vi "SpectrometerSpinCoater_v05.vi"() -> ()   [LabVIEW 2018]
uses:
  <instrlib>/Classes/CCD/Abstract_CCD/Abstract_CCD.lvclass
  TypDef/DeviceQueue_Action.ctl
  TypDef/DeviceQueue_TypeDef.ctl
  TypDef/DataQueue_Action.ctl
  TypDef/DataQueue_TypeDef.ctl
  <instrlib>/Classes/CCD/Avantes/Avantes.lvclass
  <vilib>/Utility/error.llb/DialogType.ctl
  <vilib>/Instr/_visa.llb/VISA Configure Serial Port (Instr).vi
  <vilib>/Analysis/NI_AALBase.lvlib
  <vilib>/Analysis/baseanly.llb/A x Vector.vi
  TypDef/TabControl.ctl
  C:/Program Files/National Instruments/LabVIEW 2018/instr.lib/Classes/CCD/Abstract_CCD/Abstract_CCD.lvclass
panel:
  out "Time.spin":refnum<file>
  out "Meas.spin":refnum<file>
  out "Arduino":bool
  out "NKT":bool
  out "Spectromter":bool
  in  "Abort Button":bool
  in  "Stop Button":bool
  in  "Tab Control":enum32{"Measure", "Settings"}(tab)=enum."Settings"
  in  "Spectra Count":u16
  in  "Measure Spectrum":bool
  out "Action":string
  in  "Preview":bool
  out "XY Graph":T1(graph)
  in  "Frames for Spectrometer":dbl=1.0
  in  "StartSpin_Button":bool
  out "Overall Time":dbl
  in  "Seconds after Spin Stop":dbl[unit]=0.5
  in  "Program Spin Coater\nSpeed (rpm)          Time (s)":dbl[][](array[numeric])
  in  "Record RefSpec":bool
  in  "Record_Darkspec":bool
  in  "Comments":string="Just for testing"
  in  "File Name":string="Temp"
  in  "Save Path":path=path "C:/Users/Timo/Desktop/SpinCoater/Measurement"
  in  "Seconds to Spin Start":dbl[unit]=1.0
  in  "Calculate Frames":bool=TRUE
  in  "Frames":i32
  out "Frame Rate":dbl[unit]
  in  "Integration Time":dbl[unit]=3e-05
  in  "StartMeasurement_Button":bool
  in  "Dividider Get Spectra":u32=1 min=1
  in  "Automatically \nadjust count":bool
  in  "Reset Count\nafter Spin Coating":bool
  in  "Speed":dbl
  in  "Milliseconds":dbl
  in  "Debug":bool
  in  "Port Arduino":refnum<visa-resource-name>="COM6"
  out "Error Arduino":bool caption="Error"
  in  "Init_Arduino":bool=TRUE caption="Init"
  out "Caption_Settings_Arduino":string="Arduino"
  out "Caption_Settings_NKT":string="NKT Laser"
  out "Error_Spectromter":bool caption="Error"
  in  "Init_Spectrometer":bool=TRUE caption="Init"
  out "Caption_Settings_Spectrometer":string="Spectromter"
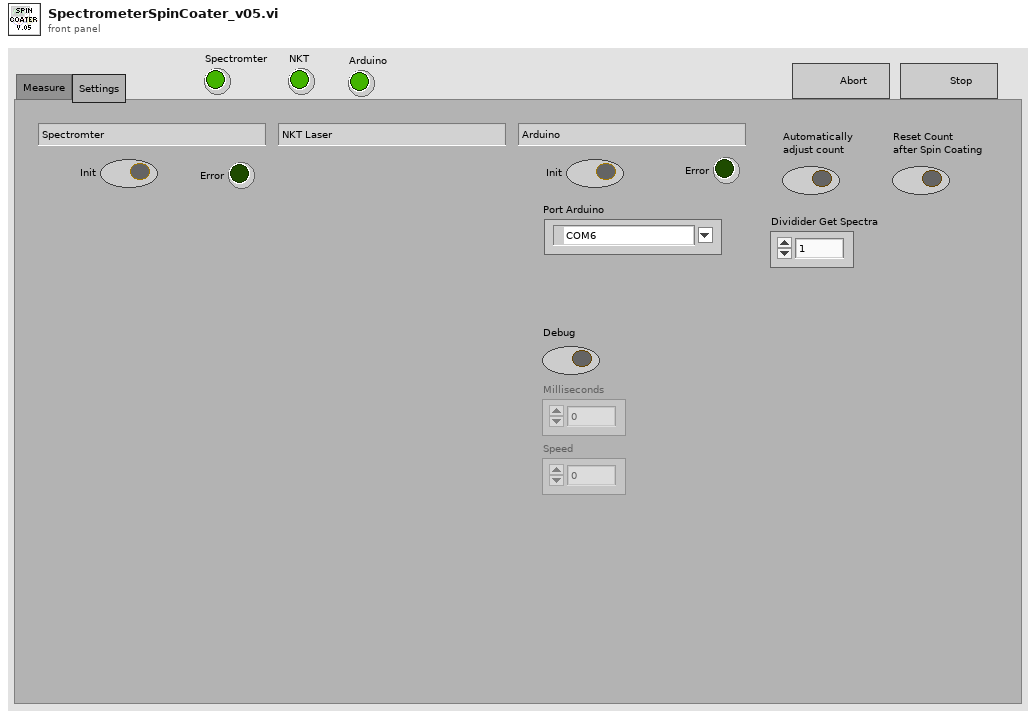
[diagram p1: front panel]
types:
  T1 = cluster{"Wavlength":dbl[unit][], "Image":dbl[]}[]
  T2 = cluster{"Dark":cluster{"Image":dbl[][][], "Frame Size":cluster{"F":i32, "Y":i32, "X":i32}}[], "Ref":cluster{"Image":dbl[][][], "Frame Size":cluster{"F":i32, "Y":i32, "X":i32}}[], "Wavlength":dbl[unit][], "spec":dbl[][]}
  T3 = cluster{"Port Arduino":refnum<visa-resource-name>, "Abstract_CCD.lvclass":refnum<class "Abstract_CCD.lvclass">}
  T4 = typedef "DataQueue_TypeDef.ctl" = cluster{"QueueAction":T5, "Data":cluster{"Image":dbl[][][], "Frame Size":cluster{"F":i32, "Y":i32, "X":i32}}[], "Data_Raw":cluster{"Image":dbl[][][], "Frame Size":cluster{"F":i32, "Y":i32, "X":i32}}[], "Data_Dark":cluster{"Image":dbl[][][], "Frame Size":cluster{"F":i32, "Y":i32, "X":i32}}[], "Data_Ref":cluster{"Image":dbl[][][], "Frame Size":cluster{"F":i32, "Y":i32, "X":i32}}[], "Device Information":string[], "Numeric Control":dbl, "Boolean":bool, "Wavelength":dbl[unit][], "Time":dbl[], "Time Stamp":timestamp, "Numeric Control 2":dbl, "TabControl":T6}
  T5 = typedef "DataQueue_Action.ctl" = enum16{"TimeOut", "Close_Program", "Abort", "Stop_Measurement", "Measure_InSituSpinCoating", "Measure_Spectrum", "Measure_SpectrumAdvanced", "Measure_SpectralStability", "Save_InSitu", "Save_SpectralStability", "Set_Ref", "Set_Dark", "Set_Wavelength", "Spectrometer_Measure", "Spectrometer_Preview", "Transfer_Settings"}
  T6 = typedef "TabControl.ctl" = enum16{"Measure", "Spectral Stability", "Settings"}
  T7 = typedef "DeviceQueue_TypeDef.ctl" = cluster{"QueueAction":T8, "Numeric 1":dbl, "Numeric 2":dbl, "Boolean 1":bool, "Boolean 2":bool, "Spin Program":dbl[][], "Spin Prg v07":cluster{"Speed (rpm)":dbl, "Time (s)":dbl, "Acc (rpm/s)":dbl}[], "Time Stamp":timestamp, "TabControl":T6}
  T8 = typedef "DeviceQueue_Action.ctl" = enum16{"TimeOut", "Wait", "Close_Program", "Abort", "Spectrometer_Init", "Spectrometer_Close", "Spectrometer_DeviceInformation", "Spectrometer_Measure", "Spectrometer_MeasureAdvanced", "Spectrometer_Preview", "Spectrometer_Abort", "Spectrometer_StartMeasurement", "Spectrometer_GetData", "Spectrometer_StopMeasurement", "Spectrometer_SetIntegrationTime", "Spectrometer_SetFrames", "Spectrometer_SetDarkspec", "Spectrometer_SetReference", "Spectrometer_SetTriggerMode", "Laser_Init", "Laser_Close", "Arduino_Init", "Arduino_Close", "Arduino_LoadProgram", "Arduino_StartProgram", "Arduino_SetSpeed", "Arduino_SetMillis", "Arduino_StopSpin", "Measure_InSitu", "Measure_Spectrum", "Measure_InSituAdvanced", "Measure_SpectralStability", "Measure_Stop"}
  T9 = typedef "DataQueue_Action.ctl" = enum16{"TimeOut", "Close_Program", "Stop_Measurement", "Measure_InSituSpinCoating", "Measure_Spectrum", "Save_Data", "Set_Ref", "Set_Dark", "Set_Wavelength", "Spectrometer_Measure", "Spectrometer_Preview", "Transfer_Settings"}
  T10 = enum16{"open", "replace", "create", "open or create", "replace or create", "replace or create with confirmation"}
  T11 = cluster{"Image":dbl[][][], "Frame Size":cluster{"F":i32, "Y":i32, "X":i32}}[]
  T12 = cluster{"Image":dbl[][][], "Frame Size":cluster{"F":i32, "Y":i32, "X":i32}}
  T13 = cluster{"Wavlength":dbl[unit][], "A x Vector":dbl[]}
  T14 = cluster{"Wavlength":dbl[unit][], "A x Vector":dbl[]}[]
  T15 = cluster{u16[][], u16[][], dbl[], "Numeric Control":dbl, "Numeric Control 2":dbl}
  T16 = typedef "DialogType.ctl" = u16
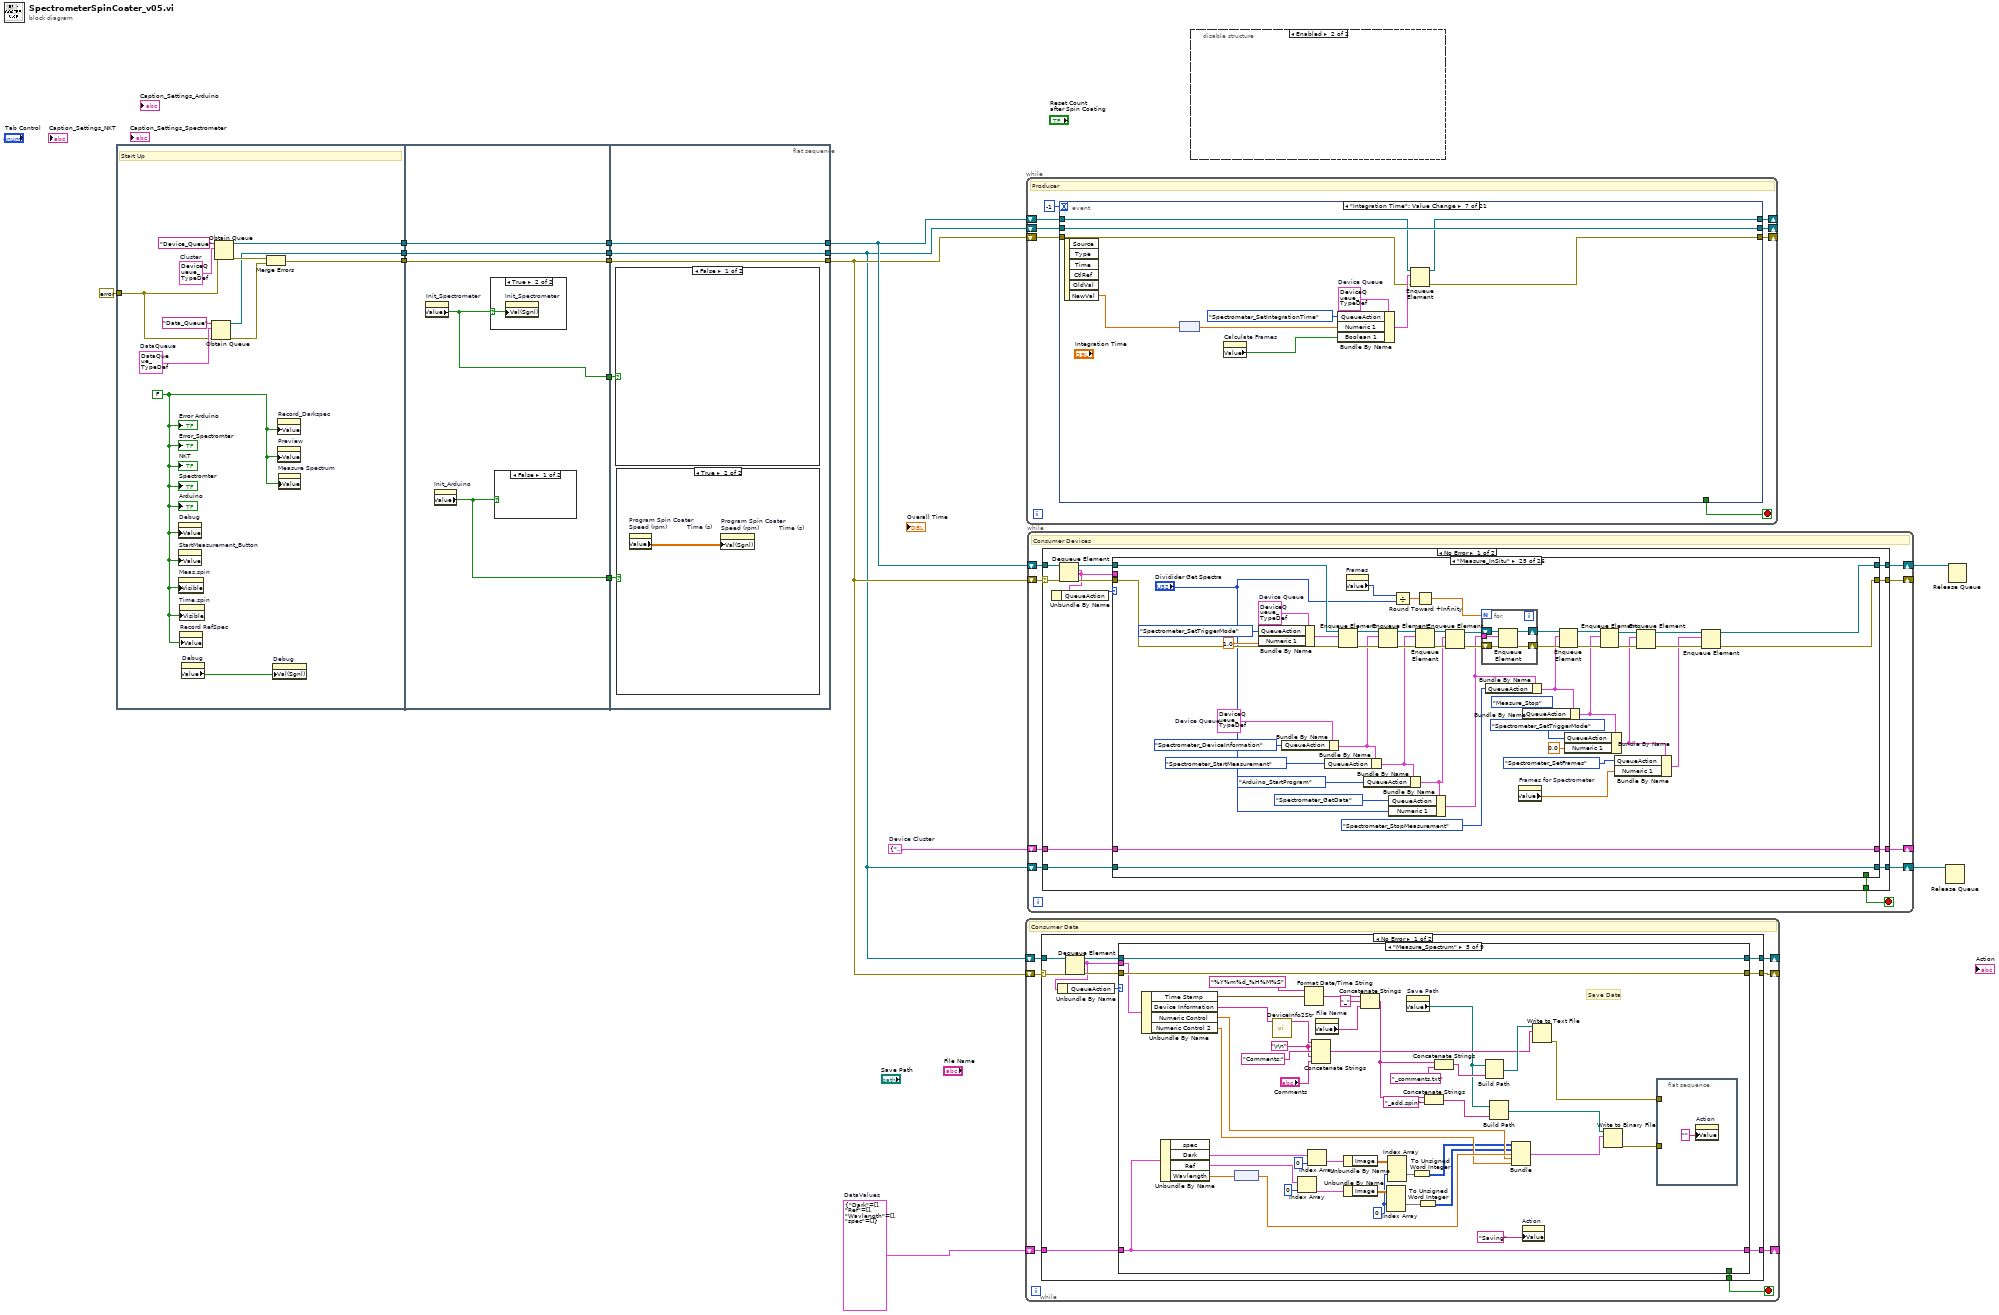
[diagram p0: block diagram]
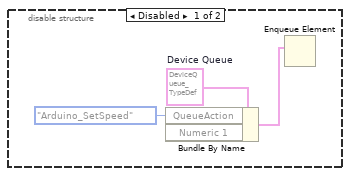
[diagram p2: hidden frame]
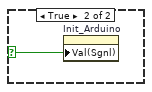
[diagram p3: hidden frame]
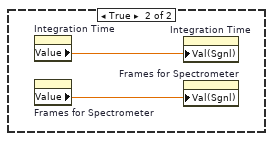
[diagram p6: hidden frame]
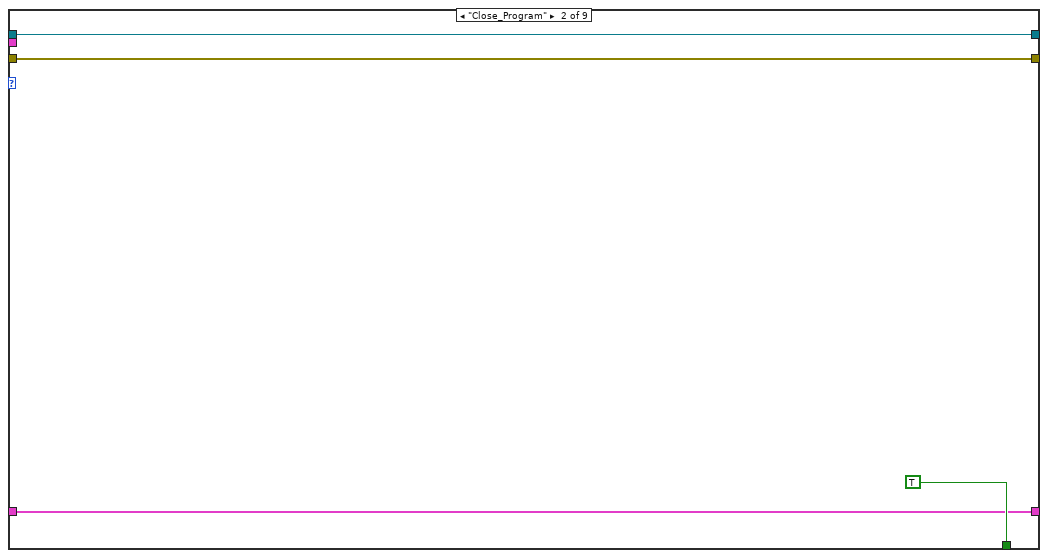
[diagram p8: hidden frame]
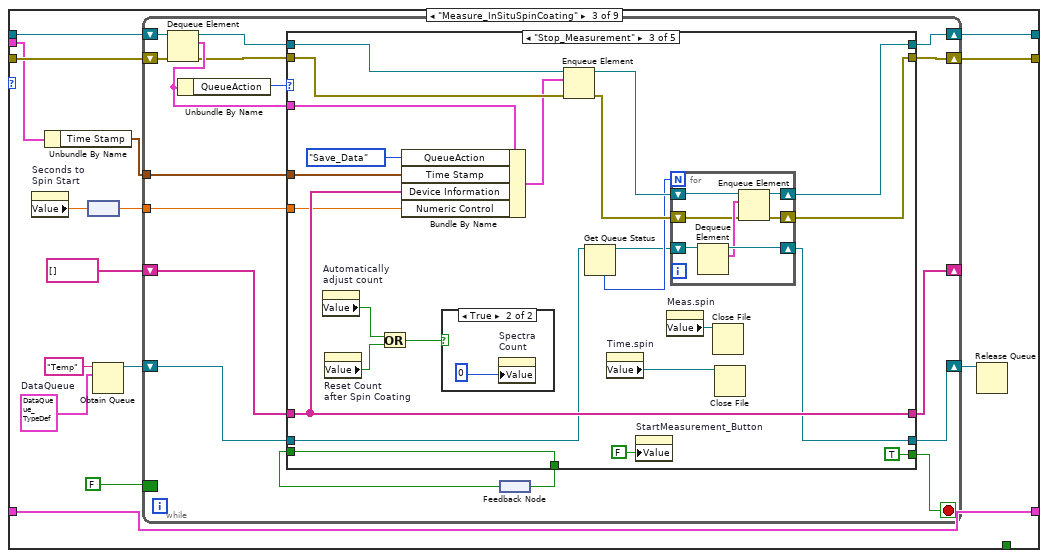
[diagram p9: hidden frame]
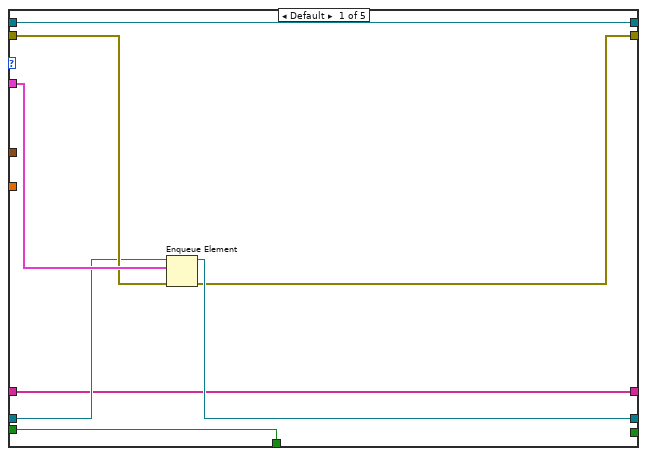
[diagram p10: hidden frame]
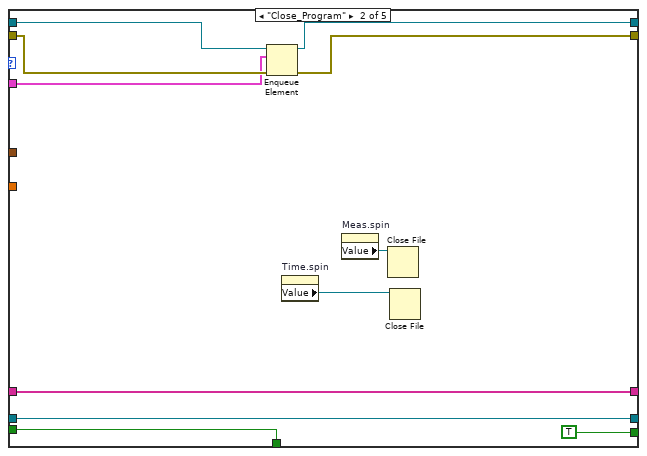
[diagram p11: hidden frame]
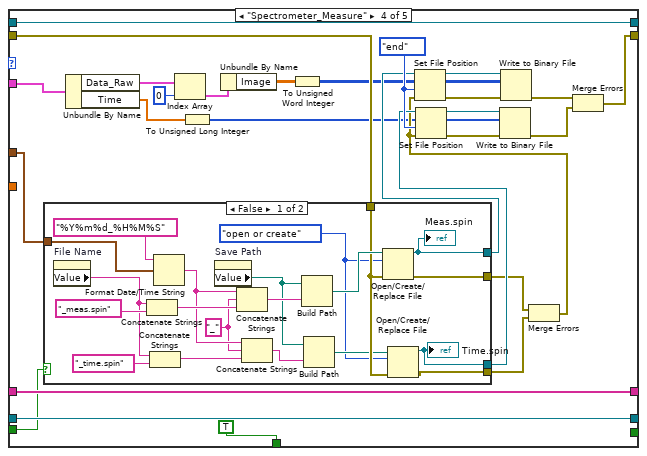
[diagram p13: hidden frame]
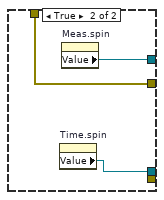
[diagram p14: hidden frame]
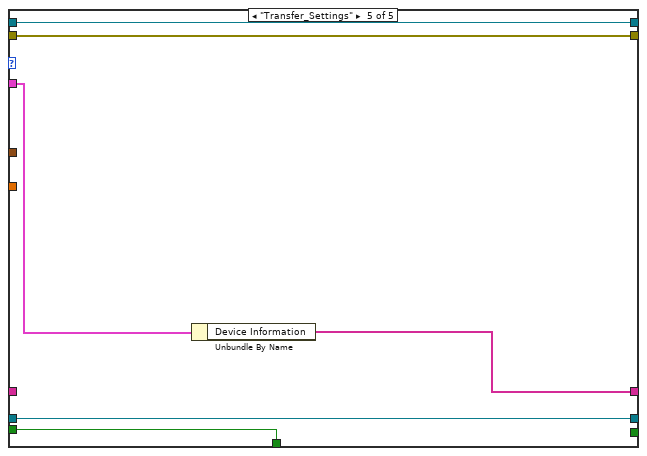
[diagram p15: hidden frame]
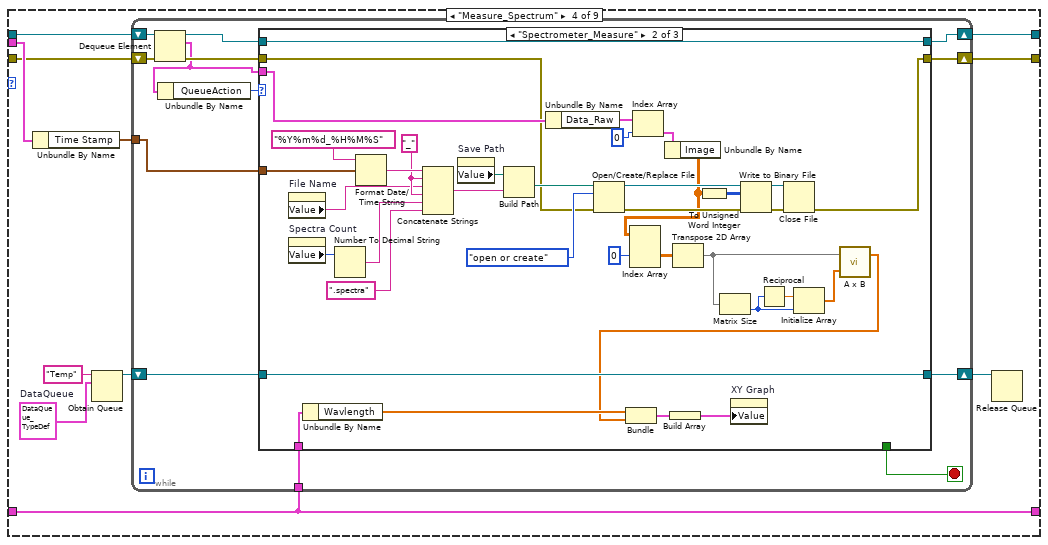
[diagram p16: hidden frame]
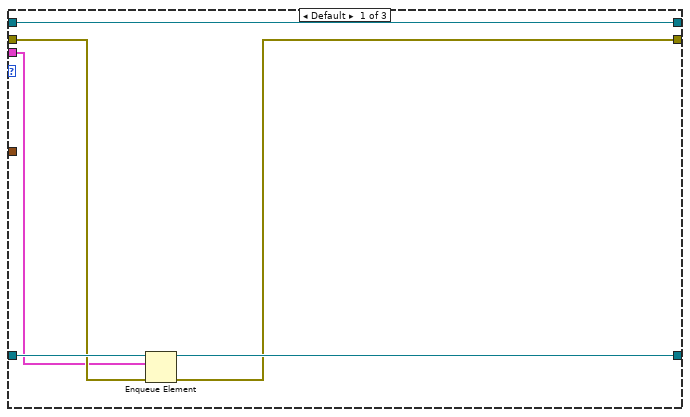
[diagram p17: hidden frame]
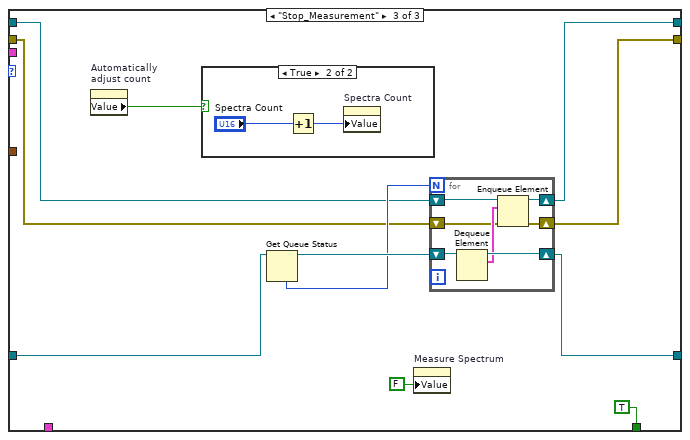
[diagram p18: hidden frame]
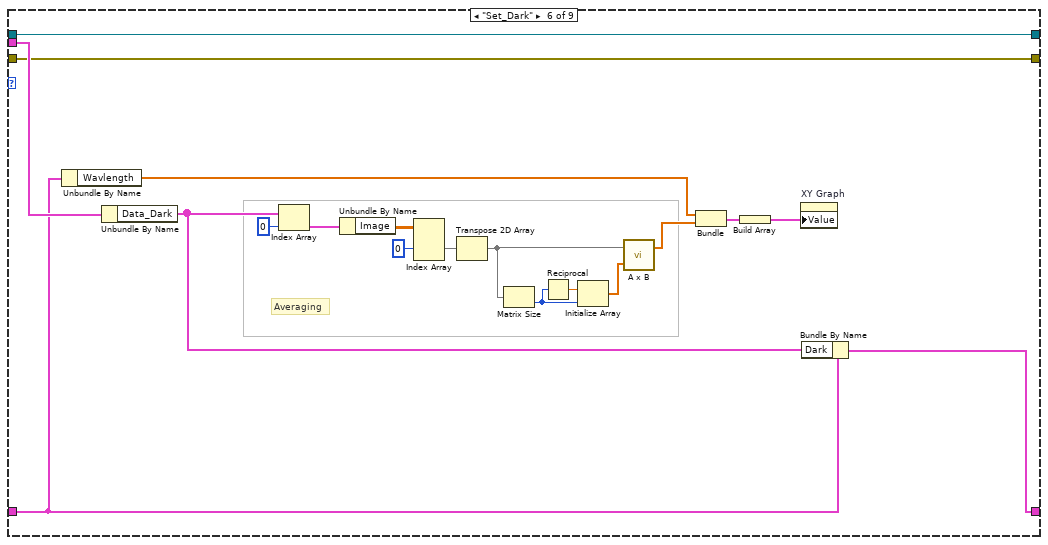
[diagram p20: hidden frame]
diagram:
  w6 = T2 {"Dark"=[], "Ref"=[], "Wavlength"=[], "spec"=[]}  # DataValues
  w11 = T3 {"Port Arduino"="", "Abstract_CCD.lvclass"=refnum}  # Device Cluster
  n1 = flat-sequence {
    tunnel: errorcluster {"status"=FALSE, "code"=0, "source"=""} ("error constant") -> [w23]
    tunnel: [w26] -> w15
    tunnel: [w20] -> w14
    tunnel: [w19] -> w13
    tunnel: w15 -> [w33]
    tunnel: w14 -> [w32]
    tunnel: w13 -> [w31]
    tunnel: [w33] -> w5
    tunnel: [w32] -> w4
    tunnel: [w31] -> w3
    tunnel: [w30] -> w2
    tunnel: [w29] -> w1
    tunnel: [w38] -> w8
    tunnel: [w39] -> w7
    tunnel: [w40] -> w12
    tunnel: w5 -> [w40]
    tunnel: w4 -> [w39]
    tunnel: w3 -> [w38]
    tunnel: w2 -> [w37]
    tunnel: w1 -> [w36]
    frame #0 {
      w24 = T4 {"QueueAction"=enum."TimeOut", "Data"=[], "Data_Raw"=[], "Data_Dark"=[], "Data_Ref"=[], "Device Information"=[], "Numeric Control"=0.0, "Boolean"=FALSE, "Wavelength"=[], "Time"=[], "Time Stamp"=timestamp(0 s since 1904-01-01), "Numeric Control 2"=0.0, "TabControl"=enum."Measure"}  # DataQueue
      w27 = T7 {"QueueAction"=enum."TimeOut", "Numeric 1"=0.0, "Numeric 2"=0.0, "Boolean 1"=FALSE, "Boolean 2"=FALSE, "Spin Program"=[], "Spin Prg v07"=[], "Time Stamp"=timestamp(0 s since 1904-01-01), "TabControl"=enum."Measure"}  # Cluster
      w18 = FALSE ("Error Arduino")
      # "Start Up"
      n2 = property on="Debug" class="Bool (strict)"("Value"=w18) -> ()  [unwired: 2 in, 2 out]
      n3 = property on="StartMeasurement_Button" class="Bool (strict)"("Value"=w18) -> ()  [unwired: 2 in, 2 out]
      n4 = property on="Meas.spin" class="Ref (strict)"("Visible"=w18) -> ()  [unwired: 2 in, 2 out]
      n5 = property on="Time.spin" class="Ref (strict)"("Visible"=w18) -> ()  [unwired: 2 in, 2 out]
      n6 = property on="Record RefSpec" class="Bool (strict)"("Value"=w18) -> ()  [unwired: 2 in, 2 out]
      n7 = property on="Debug" class="Bool (strict)"() -> ("Value"=w17:bool)  [unwired: 2 in, 2 out]
      n8 = Obtain Queue(name (unnamed)="Data_Queue", element data type=w24, error in (no error)=w23) -> (queue out=w20:refnum<queue>, error out=w21:errorcluster)  [unwired: 2 in, 1 out]
      n9 = Obtain Queue(name (unnamed)="Device_Queue", element data type=w27, error in (no error)=w23) -> (queue out=w26:refnum<queue>, error out=w22:errorcluster)  [unwired: 2 in, 1 out]
      n10 = Merge Errors(w22, w21) -> (w19:errorcluster)
      n11 = property on="Debug" class="Bool (strict)"("Val(Sgnl)"=w17) -> ()  [unwired: 2 in, 2 out]
      n12 = property on="Record_Darkspec" class="Bool (strict)"("Value"=w18) -> ()  [unwired: 2 in, 2 out]
      n13 = property on="Preview" class="Bool (strict)"("Value"=w18) -> ()  [unwired: 2 in, 2 out]
      n14 = property on="Measure Spectrum" class="Bool (strict)"("Value"=w18) -> ()  [unwired: 2 in, 2 out]
      "Error_Spectromter" <- w18
      "Error Arduino" <- w18
      "Spectromter" <- w18
      "NKT" <- w18
      "Arduino" <- w18
    }
    frame #1 {
      n15 = property on="Init_Spectrometer" class="Bool (strict)"() -> ("Value"=w30:bool)  [unwired: 2 in, 2 out]
      n16 = property on="Init_Arduino" class="Bool (strict)"() -> ("Value"=w29:bool)  [unwired: 2 in, 2 out]
      n17 = case shown="True" w30 {
        selector: w30 -> [_ w35]
        frame False {
        }
        frame True {
          n18 = property on="Init_Spectrometer" class="Bool (strict)"("Val(Sgnl)"=w35) -> ()  [unwired: 2 in, 2 out]
        }
      }
      n19 = case shown="False" w29 {
        selector: w29 -> [_ w34]
        frame False {
        }
        frame True {
          n20 = property on="Init_Arduino" class="Bool (strict)"("Val(Sgnl)"=w34) -> ()  [unwired: 2 in, 2 out]
        }
      }
    }
    frame #2 {
      n21 = case shown="False" w37 {
        frame False {
        }
        frame True {
          n22 = property on="Integration Time" class="DigNum (strict)"() -> ("Value"=w42:dbl[unit])  [unwired: 2 in, 2 out]
          n23 = property on="Frames for Spectrometer" class="DigNum (strict)"() -> ("Value"=w43:dbl)  [unwired: 2 in, 2 out]
          n24 = property on="Integration Time" class="DigNum (strict)"("Val(Sgnl)"=w42) -> ()  [unwired: 2 in, 2 out]
          n25 = property on="Frames for Spectrometer" class="DigNum (strict)"("Val(Sgnl)"=w43) -> ()  [unwired: 2 in, 2 out]
        }
      }
      n26 = case shown="True" w36 {
        frame False {
        }
        frame True {
          n27 = property on="Program Spin Coater\nSpeed (rpm)          Time (s)" class="Arr (strict)"() -> ("Value"=w41:dbl[][])  [unwired: 2 in, 2 out]
          n28 = property on="Program Spin Coater\nSpeed (rpm)          Time (s)" class="Arr (strict)"("Val(Sgnl)"=w41) -> ()  [unwired: 2 in, 2 out]
        }
      }
    }
  }
  n29 = while {
    shift-right: [w44] -> _
    shift-left: w8 -> [w50]
    shift-right: [w45] -> _
    shift-left: w7 -> [w49]
    shift-right: [w46] -> _
    shift-left: w6 -> [w48]
    stop <- w47 stop-if-true
    # "Consumer Data"
    n30 = case shown="No Error" w50 {
      selector: w50 -> [w61 w400]
      tunnel: w49 -> [w60 w401]
      tunnel: w48 -> [w58 w398]
      tunnel: [w57 _] -> w47
      tunnel: [w56 w398] -> w46
      tunnel: [w55 w401] -> w45
      tunnel: [w53 w399] -> w44
      frame No Error {
        n31 = Dequeue Element(queue=w60, error in (no error)=w61) -> (queue out=w54:refnum<queue>, element=w51:T4, error out=w52:errorcluster)  [unwired: 1 in, 1 out]
        n32 = Unbundle By Name(w51) -> ("QueueAction"=w59:T5)
        n33 = case shown="\"Measure_Spectrum\"" w59 {
          tunnel: w58 -> [w62 w67 w73 w209 w309 w352 w361 w383 w394]
          tunnel: [_ TRUE _ _ _ _ _ _ _] -> w57
          tunnel: [w62 w67 w73 w209 w309 w356 w375 w382 w394] -> w56
          tunnel: [w64 w66 w83 w215 w339 w357 w376 w379 w397] -> w55
          tunnel: w54 -> [w64 w66 w81 w217 w339 w357 w376 w379 w397]
          tunnel: [w63 w65 w82 w214 w338 w358 w377 w380 w396] -> w53
          tunnel: w52 -> [w63 w65 w80 w218 w338 w358 w377 w380 w396]
          tunnel: w51 -> [_ _ w75 w219 w325 w359 w378 w381 w395]
          frame "TimeOut", Default {
          }
          frame "Close_Program" {
          }
          frame "Measure_InSituSpinCoating" {
            w78 = T4 {"QueueAction"=enum."TimeOut", "Data"=[], "Data_Raw"=[], "Data_Dark"=[], "Data_Ref"=[], "Device Information"=[], "Numeric Control"=0.0, "Boolean"=FALSE, "Wavelength"=[], "Time"=[], "Time Stamp"=timestamp(0 s since 1904-01-01), "Numeric Control 2"=0.0, "TabControl"=enum."Measure"}  # DataQueue
            n34 = property on="Seconds to\nSpin Start" class="DigNum (strict)"() -> ("Value"=w70:dbl[unit])  [unwired: 2 in, 2 out]
            n35 = Unbundle By Name(w75) -> ("Time Stamp"=w74:timestamp)
            n36 = node(w70) -> (w69:dbl)
            n37 = Obtain Queue(name (unnamed)="Temp", element data type=w78) -> (queue out=w77:refnum<queue>)  [unwired: 3 in, 2 out]
            n38 = while {
              shift-right: [w91] -> w83
              shift-left: w81 -> [w100]
              shift-right: [w92] -> w82
              shift-left: w80 -> [w99]
              shift-right: [w93] -> w76
              shift-left: w77 -> [w94]
              tunnel: w74 -> [w87]
              shift-right: [w88] -> _
              shift-left: string[] [] ("Device Information") -> [w89]
              border: FALSE -> [_]
              tunnel: w69 -> [w84]
              stop <- w90 stop-if-true
              n39 = Dequeue Element(queue=w100, error in (no error)=w99) -> (queue out=w95:refnum<queue>, element=w97:T4, error out=w96:errorcluster)  [unwired: 1 in, 1 out]
              n40 = Unbundle By Name(w97) -> ("QueueAction"=w98:T5)
              n41 = feedback #1() -> (w86:bool)
              n42 = case shown="\"Stop_Measurement\"" w98 {
                tunnel: w97 -> [w108 w117 w142 w178 w207]
                tunnel: w96 -> [w107 w118 w139 w168 w204]
                tunnel: w95 -> [w103 w119 w138 w177 w205]
                tunnel: w94 -> [w106 w114 w133 w165 w208]
                tunnel: [w105 w114 w130 w165 w208] -> w93
                tunnel: [w104 w115 w129 w166 w204] -> w92
                tunnel: [w103 w116 w128 w177 w205] -> w91
                tunnel: [_ TRUE TRUE _ _] -> w90
                tunnel: w89 -> [w102 w112 w140 w163 _]
                tunnel: [w102 w112 w140 w163 w206] -> w88
                tunnel: w87 -> [_ _ w141 w179 _]
                tunnel: w86 -> [w101 w111 w127 w161 w203]
                tunnel: [w101 w111 w127 TRUE w203] -> w85
                tunnel: w84 -> [_ _ w124 _ _]
                frame Default {
                  n43 = Enqueue Element(queue=w106, element=w108, error in (no error)=w107) -> (queue out=w105:refnum<queue>, error out=w104:errorcluster)  [unwired: 1 in, 1 out]
                }
                frame "Close_Program" {
                  n44 = Enqueue Element(queue=w119, element=w117, error in (no error)=w118) -> (queue out=w116:refnum<queue>, error out=w115:errorcluster)  [unwired: 1 in, 1 out]
                  n45 = property on="Time.spin" class="Ref (strict)"() -> ("Value"=w109:refnum<file>)  [unwired: 2 in, 2 out]
                  n46 = property on="Meas.spin" class="Ref (strict)"() -> ("Value"=w110:refnum<file>)  [unwired: 2 in, 2 out]
                  n47 = Close File(refnum=w110) -> ()  [unwired: 1 in, 2 out]
                  n48 = Close File(refnum=w109) -> ()  [unwired: 1 in, 2 out]
                }
                frame "Stop_Measurement" {
                  n49 = property on="Automatically \nadjust count" class="Bool (strict)"() -> ("Value"=w121:bool)  [unwired: 2 in, 2 out]
                  n50 = property on="Reset Count\nafter Spin Coating" class="Bool (strict)"() -> ("Value"=w122:bool)  [unwired: 2 in, 2 out]
                  n51 = Or(x=w121, y=w122) -> (x .or. y?=w120:bool)
                  n52 = Bundle By Name(cluster=w142, "QueueAction"=DataQueue_Action."Save_Data", "Time Stamp"=w141, "Device Information"=w140, "Numeric Control"=w124) -> (w137:T4)
                  n53 = case shown="True" w120 {
                    frame False {
                    }
                    frame True {
                      n54 = property on="Spectra \nCount" class="DigNum (strict)"("Value"=u16 0 ("Spectra Count")) -> ()  [unwired: 2 in, 2 out]
                    }
                  }
                  n55 = Enqueue Element(queue=w138, element=w137, error in (no error)=w139) -> (queue out=w135:refnum<queue>, error out=w134:errorcluster)  [unwired: 1 in, 1 out]
                  n56 = Get Queue Status(queue=w133) -> (queue out=w131:refnum<queue>, # elements in queue=w132:i32)  [unwired: 2 in, 6 out]
                  n57 = property on="Time.spin" class="Ref (strict)"() -> ("Value"=w125:refnum<file>)  [unwired: 2 in, 2 out]
                  n58 = property on="StartMeasurement_Button" class="Bool (strict)"("Value"=FALSE ("StartMeasurement_Button")) -> ()  [unwired: 2 in, 2 out]
                  n59 = property on="Meas.spin" class="Ref (strict)"() -> ("Value"=w126:refnum<file>)  [unwired: 2 in, 2 out]
                  n60 = for {
                    N: w132 -> [_]
                    shift-right: [w150] -> w130
                    shift-left: w131 -> [w151]
                    shift-right: [w147] -> w128
                    shift-left: w135 -> [w148]
                    shift-right: [w145] -> w129
                    shift-left: w134 -> [w146]
                    n61 = Dequeue Element(queue=w151) -> (queue out=w150:refnum<queue>, element=w149:T4)  [unwired: 2 in, 2 out]
                    n62 = Enqueue Element(queue=w148, element=w149, error in (no error)=w146) -> (queue out=w147:refnum<queue>, error out=w145:errorcluster)  [unwired: 1 in, 1 out]
                  }
                  n63 = Close File(refnum=w126) -> ()  [unwired: 1 in, 2 out]
                  n64 = Close File(refnum=w125) -> ()  [unwired: 1 in, 2 out]
                }
                frame "Spectrometer_Measure" {
                  w164 = enum16{"start", "end", "current"}."end" ("from (0:start)")
                  n65 = case shown="False" w161 {
                    tunnel: w179 -> [w196 _]
                    tunnel: w168 -> [w191 w202]
                    tunnel: [w184 w202] -> w155
                    tunnel: [w183 _] -> w156
                    tunnel: [w182 w201] -> w158
                    tunnel: [w181 w200] -> w157
                    frame False {
                      w185 = T10."open or create" ("operation (0:open)")
                      w180 = "_" ("string")
                      n66 = property on="File Name" class="Str"() -> ("Value"=w194:string)  [unwired: 2 in, 2 out]
                      n67 = Concatenate Strings(w194, "_meas.spin" ("string")) -> (w197:string)
                      n68 = Concatenate Strings(w194, "_time.spin" ("string")) -> (w189:string)
                      n69 = Format Date/Time String(time format string (%c)="%Y%m%d_%H%M%S", seconds (now)=w196) -> (date/time string=w190:string)  [unwired: 1 in]
                      n70 = property on="Save Path" class="Path"() -> ("Value"=w187:path)  [unwired: 2 in, 2 out]
                      n71 = Concatenate Strings(w190, w180, w197) -> (w195:string)
                      n72 = Concatenate Strings(w190, w180, w189) -> (w188:string)
                      n73 = Build Path(base path=w187, name or relative path=w195) -> (appended path=w192:path)
                      n74 = Build Path(base path=w187, name or relative path=w188) -> (appended path=w186:path)
                      n75 = Open/Create/Replace File(file path (use dialog)=w192, error in=w191, operation (0:open)=w185) -> (refnum out=w182:refnum<file>, error out=w184:errorcluster)  [unwired: 3 in, 1 out]
                      "Meas.spin" <- w182
                      n76 = Open/Create/Replace File(file path (use dialog)=w186, error in=w191, operation (0:open)=w185) -> (refnum out=w181:refnum<file>, error out=w183:errorcluster)  [unwired: 3 in, 1 out]
                      "Time.spin" <- w181
                    }
                    frame True {
                      n77 = property on="Time.spin" class="Ref (strict)"() -> ("Value"=w200:refnum<file>)  [unwired: 2 in, 2 out]
                      n78 = property on="Meas.spin" class="Ref (strict)"() -> ("Value"=w201:refnum<file>)  [unwired: 2 in, 2 out]
                    }
                  }
                  n79 = Unbundle By Name(w178) -> ("Data_Raw"=w174:T11, "Time"=w167:dbl[])
                  n80 = Index Array(array=w174, index=0) -> (element=w173:T12)
                  n81 = To Unsigned Long Integer(number=w167) -> (unsigned 32bit integer=w153:u32[])
                  n82 = Unbundle By Name(w173) -> ("Image"=w171:dbl[][][])
                  n83 = To Unsigned Word Integer(number=w171) -> (unsigned 16bit integer=w152:u16[][][])
                  n84 = Merge Errors(w155, w156) -> (w154:errorcluster)
                  n85 = Set File Position(refnum=w158, from (0:start)=w164, error in=w154) -> (refnum out=w170:refnum<file>, error out=w169:errorcluster)  [unwired: 1 in]
                  n86 = Set File Position(refnum=w157, from (0:start)=w164, error in=w154) -> (refnum out=w176:refnum<file>, error out=w175:errorcluster)  [unwired: 1 in]
                  n87 = Write to Binary File(file (use dialog)=w176, data=w153, error in=w175) -> (error out=w159:errorcluster)  [unwired: 3 in, 2 out]
                  n88 = Write to Binary File(file (use dialog)=w170, data=w152, error in=w169) -> (error out=w160:errorcluster)  [unwired: 3 in, 2 out]
                  n89 = Merge Errors(w160, w159) -> (w166:errorcluster)
                }
                frame "Transfer_Settings" {
                  n90 = Unbundle By Name(w207) -> ("Device Information"=w206:string[])
                }
              }
              n91 = feedback-in #1(w85) -> ()
            }
            n92 = Release Queue(queue=w76) -> ()  [unwired: 2 in, 3 out]
          }
          frame "Measure_Spectrum" {
            w212 = T4 {"QueueAction"=enum."TimeOut", "Data"=[], "Data_Raw"=[], "Data_Dark"=[], "Data_Ref"=[], "Device Information"=[], "Numeric Control"=0.0, "Boolean"=FALSE, "Wavelength"=[], "Time"=[], "Time Stamp"=timestamp(0 s since 1904-01-01), "Numeric Control 2"=0.0, "TabControl"=enum."Measure"}  # DataQueue
            n93 = Unbundle By Name(w219) -> ("Time Stamp"=w216:timestamp)
            n94 = Obtain Queue(name (unnamed)="Temp", element data type=w212) -> (queue out=w211:refnum<queue>)  [unwired: 3 in, 2 out]
            n95 = while {
              shift-right: [w223] -> w215
              shift-left: w217 -> [w231]
              shift-right: [w224] -> w214
              shift-left: w218 -> [w232]
              tunnel: w216 -> [w221]
              shift-right: [w225] -> w210
              shift-left: w211 -> [w227]
              tunnel: w209 -> [w220]
              stop <- w222 stop-if-true
              n96 = Dequeue Element(queue=w231, error in (no error)=w232) -> (queue out=w229:refnum<queue>, element=w226:T4, error out=w228:errorcluster)  [unwired: 1 in, 1 out]
              n97 = Unbundle By Name(w226) -> ("QueueAction"=w230:T5)
              n98 = case shown="\"Spectrometer_Measure\"" w230 {
                tunnel: w229 -> [w233 w251 w282]
                tunnel: w228 -> [w236 w261 w281]
                tunnel: w227 -> [w238 w273 w284]
                tunnel: w226 -> [w234 w275 _]
                tunnel: [w237 w273 w280] -> w225
                tunnel: [w235 w252 w278] -> w224
                tunnel: [w233 w251 w279] -> w223
                tunnel: [_ _ TRUE] -> w222
                tunnel: w221 -> [_ w272 _]
                tunnel: w220 -> [_ w243 _]
                frame Default {
                  n99 = Enqueue Element(queue=w238, element=w234, error in (no error)=w236) -> (queue out=w237:refnum<queue>, error out=w235:errorcluster)  [unwired: 1 in, 1 out]
                }
                frame "Spectrometer_Measure" {
                  w269 = "_"
                  n100 = property on="File Name" class="Str"() -> ("Value"=w268:string)  [unwired: 2 in, 2 out]
                  n101 = property on="Spectra Count" class="DigNum (strict)"() -> ("Value"=w274:u16)  [unwired: 2 in, 2 out]
                  n102 = Unbundle By Name(w243) -> ("Wavlength"=w240:dbl[unit][])
                  n103 = Number To Decimal String(number=w274) -> (decimal integer string=w267:string)  [unwired: 1 in]
                  n104 = Format Date/Time String(time format string (%c)="%Y%m%d_%H%M%S", seconds (now)=w272) -> (date/time string=w270:string)  [unwired: 1 in]
                  n105 = Concatenate Strings(w270, w269, w268, w269, w267, ".spectra" ("string")) -> (w265:string)
                  n106 = property on="Save Path" class="Path"() -> ("Value"=w264:path)  [unwired: 2 in, 2 out]
                  n107 = Build Path(base path=w264, name or relative path=w265) -> (appended path=w263:path)
                  n108 = Unbundle By Name(w275) -> ("Data_Raw"=w258:T11)
                  n109 = Open/Create/Replace File(file path (use dialog)=w263, error in=w261, operation (0:open)=T10."open or create") -> (refnum out=w260:refnum<file>, error out=w259:errorcluster)  [unwired: 3 in, 1 out]
                  n110 = Index Array(array=w258, index=0) -> (element=w256:T12)
                  n111 = Unbundle By Name(w256) -> ("Image"=w244:dbl[][][])
                  n112 = Index Array(array=w244, index (dim 1)=0 ("disabled index (row)")) -> (element=w250:dbl[][])  [unwired: 2 in]
                  n113 = Transpose 2D Array(2D array=w250) -> (transposed array=w247:dbl[][])
                  n114 = To Unsigned Word Integer(number=w244) -> (unsigned 16bit integer=w255:u16[][][])
                  n115 = Matrix Size(0:w247) -> (2:w248:i32)  [unwired: 1 out]
                  n116 = Write to Binary File(file (use dialog)=w260, data=w255, error in=w259) -> (refnum out=w253:refnum<file>, error out=w254:errorcluster)  [unwired: 3 in, 1 out]
                  n117 = Reciprocal(x=w248) -> (1/x=w249:dbl)
                  n118 = Close File(refnum=w253, error in=w254) -> (error out=w252:errorcluster)  [unwired: 1 out]
                  n119 = Initialize Array(w249, w248) -> (w246:dbl[])
                  n120 = call-poly <vilib>:"A x B.vi"("Vector"=w246, "A"=w247) -> ("A x Vector"=w239:dbl[])  [unwired: 1 out]
                  n121 = Bundle("Wavlength"=w240, "A x Vector"=w239) -> (w242:T13)  [unwired: 1 in]
                  n122 = Build Array(w242) -> (w241:T14)
                  n123 = property on="XY Graph" class="XYGraph (strict)"("Value"=w241) -> ()  [unwired: 2 in, 2 out]
                }
                frame "Stop_Measurement" {
                  n124 = property on="Automatically \nadjust count" class="Bool (strict)"() -> ("Value"=w276:bool)  [unwired: 2 in, 2 out]
                  n125 = case shown="True" w276 {
                    frame False {
                    }
                    frame True {
                      n126 = Increment(x="Spectra Count") -> (x+1=w287:u16)
                      n127 = property on="Spectra Count" class="DigNum (strict)"("Value"=w287) -> ()  [unwired: 2 in, 2 out]
                    }
                  }
                  n128 = Get Queue Status(queue=w284) -> (queue out=w285:refnum<queue>, # elements in queue=w283:i32)  [unwired: 2 in, 6 out]
                  n129 = property on="Measure Spectrum" class="Bool (strict)"("Value"=FALSE ("Measure Spectrum")) -> ()  [unwired: 2 in, 2 out]
                  n130 = for {
                    N: w283 -> [_]
                    shift-right: [w294] -> w280
                    shift-left: w285 -> [w295]
                    shift-right: [w291] -> w279
                    shift-left: w282 -> [w292]
                    shift-right: [w289] -> w278
                    shift-left: w281 -> [w290]
                    n131 = Dequeue Element(queue=w295) -> (queue out=w294:refnum<queue>, element=w293:T4)  [unwired: 2 in, 2 out]
                    n132 = Enqueue Element(queue=w292, element=w293, error in (no error)=w290) -> (queue out=w291:refnum<queue>, error out=w289:errorcluster)  [unwired: 1 in, 1 out]
                  }
                }
              }
            }
            n133 = Release Queue(queue=w210) -> ()  [unwired: 2 in, 3 out]
          }
          frame "Measure_Spectrum" {
            w311 = "\r\n"
            w298 = 0 ("index (page)")
            # "Save Data"
            n134 = Unbundle By Name(w325) -> ("Time Stamp"=w323:timestamp, "Device Information"=w314:string[], "Numeric Control"=w308:dbl, "Numeric Control 2"=w307:dbl)
            n135 = Unbundle By Name(w309) -> ("Dark"=w335:T11, "Ref"=w333:T11, "Wavlength"=w337:dbl[unit][])  [unwired: 1 out]
            n136 = node(w337) -> (w326:dbl[])
            n137 = call "DeviceInfo2Str.vi"("Device Information"=w314) -> ("String"=w313:string)  [unwired: 10 in]
            n138 = Index Array(array=w333, index=0) -> (element=w331:T12)
            n139 = Format Date/Time String(time format string (%c)="%Y%m%d_%H%M%S", seconds (now)=w323) -> (date/time string=w322:string)  [unwired: 1 in]
            n140 = Index Array(array=w335, index=0) -> (element=w332:T12)
            n141 = Concatenate Strings(w313, w311, "Comments:" ("string"), w311, "Comments") -> (w306:string)
            n142 = property on="File Name" class="Str"() -> ("Value"=w304:string)  [unwired: 2 in, 2 out]
            n143 = Unbundle By Name(w332) -> ("Image"=w330:dbl[][][])
            n144 = Unbundle By Name(w331) -> ("Image"=w329:dbl[][][])
            n145 = Concatenate Strings(w322, "_" ("string"), w304) -> (w320:string)
            n146 = Index Array(array=w329, index (dim 1)=w298) -> (element=w327:dbl[][])  [unwired: 2 in]
            n147 = Index Array(array=w330, index (dim 1)=w298) -> (element=w328:dbl[][])  [unwired: 2 in]
            n148 = property on="Save Path" class="Path"() -> ("Value"=w303:path)  [unwired: 2 in, 2 out]
            n149 = To Unsigned Word Integer(number=w328) -> (unsigned 16bit integer=w297:u16[][])
            n150 = To Unsigned Word Integer(number=w327) -> (unsigned 16bit integer=w296:u16[][])
            n151 = Concatenate Strings(w320, "_add.spin" ("string")) -> (w318:string)
            n152 = Concatenate Strings(w320, "_comments.txt" ("string")) -> (w317:string)
            n153 = Build Path(base path=w303, name or relative path=w317) -> (appended path=w316:path)
            n154 = Build Path(base path=w303, name or relative path=w318) -> (appended path=w302:path)
            n155 = Bundle(w297, w296, w326, "Numeric Control"=w308, "Numeric Control 2"=w307) -> (w301:T15)  [unwired: 1 in]
            n156 = property on="Action" class="Str"("Value"="Saving" ("Action")) -> ()  [unwired: 2 in, 2 out]
            n157 = Write to Text File(file (use dialog)=w316, text=w306) -> (error out=w300:errorcluster)  [unwired: 2 in, 2 out]
            n158 = Write to Binary File(file (use dialog)=w302, data=w301) -> (error out=w299:errorcluster)  [unwired: 4 in, 2 out]
            n159 = flat-sequence {
              tunnel: w300 -> [_]
              tunnel: w299 -> [_]
              frame #0 {
                n160 = property on="Action" class="Str"("Value"="" ("Action")) -> ()  [unwired: 2 in, 2 out]
              }
            }
          }
          frame "Set_Dark" {
            # "Averaging"
            n161 = Unbundle By Name(w352) -> ("Wavlength"=w351:dbl[unit][])
            n162 = Unbundle By Name(w359) -> ("Data_Dark"=w349:T11)
            n163 = Index Array(array=w349, index=0) -> (element=w354:T12)
            n164 = Unbundle By Name(w354) -> ("Image"=w348:dbl[][][])
            n165 = Index Array(array=w348, index (dim 1)=0 ("disabled index (row)")) -> (element=w346:dbl[][])  [unwired: 2 in]
            n166 = Transpose 2D Array(2D array=w346) -> (transposed array=w343:dbl[][])
            n167 = Matrix Size(0:w343) -> (2:w344:i32)  [unwired: 1 out]
            n168 = Reciprocal(x=w344) -> (1/x=w345:dbl)
            n169 = Initialize Array(w345, w344) -> (w342:dbl[])
            n170 = call-poly <vilib>:"A x B.vi"("Vector"=w342, "A"=w343) -> ("A x Vector"=w341:dbl[])  [unwired: 1 out]
            n171 = Bundle("Wavlength"=w351, "A x Vector"=w341) -> (w353:T13)  [unwired: 1 in]
            n172 = Build Array(w353) -> (w350:T14)
            n173 = property on="XY Graph" class="XYGraph (strict)"("Value"=w350) -> ()  [unwired: 2 in, 2 out]
            n174 = Bundle By Name(cluster=w352, "Dark"=w349) -> (w356:T2)
          }
          frame "Set_Ref" {
            # "Averaging"
            n175 = Unbundle By Name(w361) -> ("Wavlength"=w360:dbl[unit][])
            n176 = Unbundle By Name(w378) -> ("Data_Ref"=w365:T11)
            n177 = Index Array(array=w365, index=0) -> (element=w373:T12)
            n178 = Unbundle By Name(w373) -> ("Image"=w372:dbl[][][])
            n179 = Index Array(array=w372, index (dim 1)=0 ("disabled index (row)")) -> (element=w370:dbl[][])  [unwired: 2 in]
            n180 = Transpose 2D Array(2D array=w370) -> (transposed array=w367:dbl[][])
            n181 = Matrix Size(0:w367) -> (2:w368:i32)  [unwired: 1 out]
            n182 = Reciprocal(x=w368) -> (1/x=w369:dbl)
            n183 = Initialize Array(w369, w368) -> (w366:dbl[])
            n184 = call-poly <vilib>:"A x B.vi"("Vector"=w366, "A"=w367) -> ("A x Vector"=w362:dbl[])  [unwired: 1 out]
            n185 = Bundle("Wavlength"=w360, "A x Vector"=w362) -> (w364:T13)  [unwired: 1 in]
            n186 = Build Array(w364) -> (w363:T14)
            n187 = Bundle By Name(cluster=w361, "Ref"=w365) -> (w375:T2)
            n188 = property on="XY Graph" class="XYGraph (strict)"("Value"=w363) -> ()  [unwired: 2 in, 2 out]
          }
          frame "Set_Wavelength" {
            n189 = Unbundle By Name(w381) -> ("Wavelength"=w384:dbl[unit][])
            n190 = Bundle By Name(cluster=w383, "Wavlength"=w384) -> (w382:T2)
          }
          frame "Spectrometer_Preview" {
            w389 = 0 ("index (page)")
            n191 = Unbundle By Name(w395) -> ("Data_Raw"=w393:T11)
            n192 = Unbundle By Name(w394) -> ("Wavlength"=w388:dbl[unit][])
            n193 = Index Array(array=w393, index=0) -> (element=w391:T12)
            n194 = Unbundle By Name(w391) -> ("Image"=w390:dbl[][][])
            n195 = Index Array(array=w390, index (dim 0)=w389, index (dim 1)=w389) -> (element=w387:dbl[])  [unwired: 1 in]
            n196 = Bundle("Wavlength"=w388, "Image"=w387) -> (w386:cluster{"Wavlength":dbl[unit][], "Image":dbl[]})  [unwired: 1 in]
            n197 = Build Array(w386) -> (→"XY Graph":T1)
          }
        }
      }
      frame Error {
        w403 = T16 4 items=["no dialog", "OK message", "continue or stop message", "OK message + warnings", "continue/stop + warnings"] ("type of dialog (OK msg:1)")
        n198 = call <vilib>:"General Error Handler.vi"("type of dialog (OK msg:1)"=w403, "error in (no error)"=w400) -> ("error out"=w402:errorcluster)  [unwired: 9 in, 4 out]
        n199 = call <vilib>:"Clear Errors.vi"("error in (no error)"=w402) -> ("error out"=w399:errorcluster)  [unwired: 5 in, 1 out]
      }
    }
  }
  n200 = while {
    shift-right: [w406] -> _
    shift-left: w12 -> [w404]
    shift-right: [w409] -> _
    shift-left: w7 -> [w410]
    shift-right: [w407] -> _
    shift-left: w8 -> [w408]
    stop <- w405 stop-if-true
    # "Producer"
    n201 = event shown="[6] \"Integration Time\": Value Change" {
      selector: _ -> [_ _ _ _ _ _ _ _ _ _ _ _ _ _ _ _ _ _ _ _ _]
      dyn-events: _ -> [_ _ _ _ _ _ _ _ _ _ _ _ _ _ _ _ _ _ _ _ _]
      timeout: -1 -> [_ _ _ _ _ _ _ _ _ _ _ _ _ _ _ _ _ _ _ _ _]
      tunnel: w410 -> [w413 w428 w432 w444 w457 w472 w484 w495 w498 w505 w524 w531 w540 w548 w563 w573 w582 w590 w595 w602 w614]
      tunnel: [w413 w425 w432 w444 w457 w472 w484 w495 w498 w505 w524 w531 w540 w547 w563 w573 w582 w590 w595 w600 w614] -> w409
      tunnel: w408 -> [w412 w427 w434 w442 w454 w471 w482 w490 w497 w502 w522 w530 w538 w554 w560 w572 w581 w589 w594 w607 w615]
      tunnel: [w412 w421 w431 w438 w453 w469 w480 w489 w497 w500 w521 w528 w537 w546 w561 w569 w578 w589 w594 w607 w615] -> w407
      tunnel: w404 -> [w414 w429 w435 w443 w456 w473 w483 w492 w499 w503 w525 w532 w541 w556 w564 w574 w583 w591 w596 w608 w613]
      tunnel: [w414 w426 w433 w439 w455 w470 w481 w491 w499 w504 w523 w529 w539 w555 w562 w570 w579 w591 w593 w606 w613] -> w406
      tunnel: [_ TRUE _ _ _ _ _ _ _ _ _ _ _ _ _ _ _ _ _ _ _] -> w405
      event Timeout {
        n202 = event-data() -> ()  [unwired: 1 in, 3 out]
      }
      event "Stop Button": Value Change {
        w417 = T4 {"QueueAction"=enum."TimeOut", "Data"=[], "Data_Raw"=[], "Data_Dark"=[], "Data_Ref"=[], "Device Information"=[], "Numeric Control"=0.0, "Boolean"=FALSE, "Wavelength"=[], "Time"=[], "Time Stamp"=timestamp(0 s since 1904-01-01), "Numeric Control 2"=0.0, "TabControl"=enum."Measure"}  # DataQueue
        w420 = T7 {"QueueAction"=enum."TimeOut", "Numeric 1"=0.0, "Numeric 2"=0.0, "Boolean 1"=FALSE, "Boolean 2"=FALSE, "Spin Program"=[], "Spin Prg v07"=[], "Time Stamp"=timestamp(0 s since 1904-01-01), "TabControl"=enum."Measure"}  # Device Queue
        n203 = event-data() -> ()  [unwired: 1 in, 6 out]
        n204 = Bundle By Name(cluster=w420, "QueueAction"=DeviceQueue_Action."Close_Program") -> (w418:T7)
        n205 = Enqueue Element(queue=w429, element=w418, error in (no error)=w427) -> (queue out=w426:refnum<queue>, error out=w422:errorcluster)  [unwired: 1 in, 1 out]
        n206 = Bundle By Name(cluster=w417, "QueueAction"=DataQueue_Action."Close_Program") -> (w415:T4)
        n207 = Enqueue Element(queue=w428, element=w415, error in (no error)=w427) -> (queue out=w425:refnum<queue>, error out=w423:errorcluster)  [unwired: 1 in, 1 out]
        n208 = Merge Errors(w423, w422) -> (w421:errorcluster)
      }
      event "Abort Button": Value Change {
        w437 = T7 {"QueueAction"=enum."TimeOut", "Numeric 1"=0.0, "Numeric 2"=0.0, "Boolean 1"=FALSE, "Boolean 2"=FALSE, "Spin Program"=[], "Spin Prg v07"=[], "Time Stamp"=timestamp(0 s since 1904-01-01), "TabControl"=enum."Measure"}  # Device Queue
        # "At the moment just spin coater in non in-situ measurements can be stopped"
        n209 = event-data() -> ()  [unwired: 1 in, 6 out]
        n210 = Bundle By Name(cluster=w437, "QueueAction"=DeviceQueue_Action."Abort") -> (w436:T7)
        n211 = Enqueue Element(queue=w435, element=w436, error in (no error)=w434) -> (queue out=w433:refnum<queue>, error out=w431:errorcluster)  [unwired: 1 in, 1 out]
      }
      event "Init_Spectrometer": Value Change {
        n212 = event-data() -> ()  [unwired: 1 in, 6 out]
        n213 = case shown="True" "Init_Spectrometer" {
          tunnel: [w445 w448] -> w440
          frame True {
            n214 = Bundle By Name(cluster=T7 {"QueueAction"=enum."TimeOut", "Numeric 1"=0.0, "Numeric 2"=0.0, "Boolean 1"=FALSE, "Boolean 2"=FALSE, "Spin Program"=[], "Spin Prg v07"=[], "Time Stamp"=timestamp(0 s since 1904-01-01), "TabControl"=enum."Measure"} ("element"), "QueueAction"=DeviceQueue_Action."Spectrometer_Init") -> (w445:T7)
          }
          frame False {
            n215 = Bundle By Name(cluster=T7 {"QueueAction"=enum."TimeOut", "Numeric 1"=0.0, "Numeric 2"=0.0, "Boolean 1"=FALSE, "Boolean 2"=FALSE, "Spin Program"=[], "Spin Prg v07"=[], "Time Stamp"=timestamp(0 s since 1904-01-01), "TabControl"=enum."Measure"} ("element"), "QueueAction"=DeviceQueue_Action."Spectrometer_Close") -> (w448:T7)
          }
        }
        n216 = Enqueue Element(queue=w443, element=w440, error in (no error)=w442) -> (queue out=w439:refnum<queue>, error out=w438:errorcluster)  [unwired: 1 in, 1 out]
      }
      event "Init_Arduino": Value Change {
        n217 = event-data() -> ("NewVal"=w452:bool)  [unwired: 1 in, 5 out]
        n218 = case shown="True" w452 {
          tunnel: [w458 w461] -> w451
          frame False {
            w460 = T7 {"QueueAction"=enum."TimeOut", "Numeric 1"=0.0, "Numeric 2"=0.0, "Boolean 1"=FALSE, "Boolean 2"=FALSE, "Spin Program"=[], "Spin Prg v07"=[], "Time Stamp"=timestamp(0 s since 1904-01-01), "TabControl"=enum."Measure"}  # Device Queue
            n219 = Bundle By Name(cluster=w460, "QueueAction"=DeviceQueue_Action."Arduino_Close") -> (w458:T7)
          }
          frame True {
            w463 = T7 {"QueueAction"=enum."TimeOut", "Numeric 1"=0.0, "Numeric 2"=0.0, "Boolean 1"=FALSE, "Boolean 2"=FALSE, "Spin Program"=[], "Spin Prg v07"=[], "Time Stamp"=timestamp(0 s since 1904-01-01), "TabControl"=enum."Measure"}  # Device Queue
            n220 = Bundle By Name(cluster=w463, "QueueAction"=DeviceQueue_Action."Arduino_Init") -> (w461:T7)
          }
        }
        n221 = Enqueue Element(queue=w456, element=w451, error in (no error)=w454) -> (queue out=w455:refnum<queue>, error out=w453:errorcluster)  [unwired: 1 in, 1 out]
      }
      event "Program Spin Coater\nSpeed (rpm)          Time (s)": Value Change {
        w475 = T7 {"QueueAction"=enum."TimeOut", "Numeric 1"=0.0, "Numeric 2"=0.0, "Boolean 1"=FALSE, "Boolean 2"=FALSE, "Spin Program"=[], "Spin Prg v07"=[], "Time Stamp"=timestamp(0 s since 1904-01-01), "TabControl"=enum."Measure"}  # Device Queue
        n222 = event-data() -> ("NewVal"=w467:dbl[][])  [unwired: 1 in, 5 out]
        n223 = property on="Seconds to Spin Start" class="DigNum (strict)"() -> ("Value"=w465:dbl[unit])  [unwired: 2 in, 2 out]
        n224 = node(w465) -> (w464:dbl)
        n225 = Bundle By Name(cluster=w475, "QueueAction"=DeviceQueue_Action."Arduino_LoadProgram", "Spin Program"=w467, "Numeric 1"=w464) -> (w474:T7)
        n226 = Enqueue Element(queue=w473, element=w474, error in (no error)=w471) -> (queue out=w470:refnum<queue>, error out=w469:errorcluster)  [unwired: 1 in, 1 out]
        n227 = property on="Integration Time" class="DigNum (strict)"() -> ("Value"=w466:dbl[unit])  [unwired: 2 in, 2 out]
        n228 = property on="Integration Time" class="DigNum (strict)"("Val(Sgnl)"=w466) -> ()  [unwired: 2 in, 2 out]
      }
      event "Integration Time": Value Change {
        w486 = T7 {"QueueAction"=enum."TimeOut", "Numeric 1"=0.0, "Numeric 2"=0.0, "Boolean 1"=FALSE, "Boolean 2"=FALSE, "Spin Program"=[], "Spin Prg v07"=[], "Time Stamp"=timestamp(0 s since 1904-01-01), "TabControl"=enum."Measure"}  # Device Queue
        n229 = event-data() -> ("NewVal"=w478:dbl[unit])  [unwired: 1 in, 5 out]
        n230 = node(w478) -> (w477:dbl)
        n231 = property on="Calculate Frames" class="Bool (strict)"() -> ("Value"=w476:bool)  [unwired: 2 in, 2 out]
        n232 = Bundle By Name(cluster=w486, "QueueAction"=DeviceQueue_Action."Spectrometer_SetIntegrationTime", "Numeric 1"=w477, "Boolean 1"=w476) -> (w485:T7)
        n233 = Enqueue Element(queue=w483, element=w485, error in (no error)=w482) -> (queue out=w481:refnum<queue>, error out=w480:errorcluster)  [unwired: 1 in, 1 out]
      }
      event "Frames": Value Change {
        w494 = T7 {"QueueAction"=enum."TimeOut", "Numeric 1"=0.0, "Numeric 2"=0.0, "Boolean 1"=FALSE, "Boolean 2"=FALSE, "Spin Program"=[], "Spin Prg v07"=[], "Time Stamp"=timestamp(0 s since 1904-01-01), "TabControl"=enum."Measure"}  # Device Queue
        n234 = event-data() -> ()  [unwired: 1 in, 6 out]
        n235 = Bundle By Name(cluster=w494, "QueueAction"=DeviceQueue_Action."Spectrometer_SetFrames", "Numeric 1"="Frames") -> (w493:T7)
        n236 = Enqueue Element(queue=w492, element=w493, error in (no error)=w490) -> (queue out=w491:refnum<queue>, error out=w489:errorcluster)  [unwired: 1 in, 1 out]
      }
      event "Seconds to Spin Start", "Seconds after Spin Stop": Value Change {
        n237 = event-data() -> ()  [unwired: 1 in, 6 out]
        n238 = property on="Program Spin Coater\nSpeed (rpm)          Time (s)" class="Arr (strict)"() -> ("Value"=w496:dbl[][])  [unwired: 2 in, 2 out]
        n239 = property on="Program Spin Coater\nSpeed (rpm)          Time (s)" class="Arr (strict)"("Val(Sgnl)"=w496) -> ()  [unwired: 2 in, 2 out]
      }
      event "Calculate Frames": Value Change {
        n240 = event-data() -> ("NewVal"=w506:bool)  [unwired: 1 in, 5 out]
        n241 = case shown="False" w506 {
          tunnel: [0 2] -> w501
          tunnel: w503 -> [w508 w517]
          tunnel: [w508 w515] -> w504
          tunnel: w502 -> [w507 w514]
          tunnel: [w507 w510] -> w500
          frame False {
          }
          frame True {
            w516 = T7 {"QueueAction"=enum."TimeOut", "Numeric 1"=0.0, "Numeric 2"=0.0, "Boolean 1"=FALSE, "Boolean 2"=FALSE, "Spin Program"=[], "Spin Prg v07"=[], "Time Stamp"=timestamp(0 s since 1904-01-01), "TabControl"=enum."Measure"}  # Device Queue
            n242 = property on="Integration Time" class="DigNum (strict)"() -> ("Value"=w512:dbl[unit])  [unwired: 2 in, 2 out]
            n243 = node(w512) -> (w511:dbl)
            n244 = Bundle By Name(cluster=w516, "QueueAction"=DeviceQueue_Action."Spectrometer_SetIntegrationTime", "Numeric 1"=w511) -> (w518:T7)
            n245 = Enqueue Element(queue=w517, element=w518, error in (no error)=w514) -> (queue out=w515:refnum<queue>, error out=w510:errorcluster)  [unwired: 1 in, 1 out]
          }
        }
        n246 = property on="Frames" class="DigNum (strict)"("DisabledEnum"=w501) -> ()  [unwired: 2 in, 2 out]
      }
      event "Record RefSpec": Value Change {
        w527 = T7 {"QueueAction"=enum."TimeOut", "Numeric 1"=0.0, "Numeric 2"=0.0, "Boolean 1"=FALSE, "Boolean 2"=FALSE, "Spin Program"=[], "Spin Prg v07"=[], "Time Stamp"=timestamp(0 s since 1904-01-01), "TabControl"=enum."Measure"}  # Device Queue
        n247 = event-data() -> ()  [unwired: 1 in, 6 out]
        n248 = Bundle By Name(cluster=w527, "QueueAction"=DeviceQueue_Action."Spectrometer_SetReference") -> (w526:T7)
        n249 = Enqueue Element(queue=w525, element=w526, error in (no error)=w522) -> (queue out=w523:refnum<queue>, error out=w521:errorcluster)  [unwired: 1 in, 1 out]
      }
      event "Preview": Value Change {
        w535 = T7 {"QueueAction"=enum."TimeOut", "Numeric 1"=0.0, "Numeric 2"=0.0, "Boolean 1"=FALSE, "Boolean 2"=FALSE, "Spin Program"=[], "Spin Prg v07"=[], "Time Stamp"=timestamp(0 s since 1904-01-01), "TabControl"=enum."Measure"}  # Device Queue
        n250 = event-data() -> ()  [unwired: 1 in, 6 out]
        n251 = Bundle By Name(cluster=w535, "QueueAction"=DeviceQueue_Action."Spectrometer_Preview") -> (w534:T7)
        n252 = Enqueue Element(queue=w532, element=w534, error in (no error)=w530) -> (queue out=w529:refnum<queue>, error out=w528:errorcluster)  [unwired: 1 in, 1 out]
      }
      event "Record_Darkspec": Value Change {
        w543 = T7 {"QueueAction"=enum."TimeOut", "Numeric 1"=0.0, "Numeric 2"=0.0, "Boolean 1"=FALSE, "Boolean 2"=FALSE, "Spin Program"=[], "Spin Prg v07"=[], "Time Stamp"=timestamp(0 s since 1904-01-01), "TabControl"=enum."Measure"}  # Device Queue
        n253 = event-data() -> ()  [unwired: 1 in, 6 out]
        n254 = Bundle By Name(cluster=w543, "QueueAction"=DeviceQueue_Action."Spectrometer_SetDarkspec") -> (w542:T7)
        n255 = Enqueue Element(queue=w541, element=w542, error in (no error)=w538) -> (queue out=w539:refnum<queue>, error out=w537:errorcluster)  [unwired: 1 in, 1 out]
      }
      event "StartMeasurement_Button": Value Change {
        w550 = T4 {"QueueAction"=enum."TimeOut", "Data"=[], "Data_Raw"=[], "Data_Dark"=[], "Data_Ref"=[], "Device Information"=[], "Numeric Control"=0.0, "Boolean"=FALSE, "Wavelength"=[], "Time"=[], "Time Stamp"=timestamp(0 s since 1904-01-01), "Numeric Control 2"=0.0, "TabControl"=enum."Measure"}  # DataQueue
        w558 = T7 {"QueueAction"=enum."TimeOut", "Numeric 1"=0.0, "Numeric 2"=0.0, "Boolean 1"=FALSE, "Boolean 2"=FALSE, "Spin Program"=[], "Spin Prg v07"=[], "Time Stamp"=timestamp(0 s since 1904-01-01), "TabControl"=enum."Measure"}  # Device Queue
        n256 = event-data() -> ()  [unwired: 1 in, 6 out]
        n257 = property on="Preview" class="Bool (strict)"("Value"=FALSE ("Preview")) -> ()  [unwired: 2 in, 2 out]
        n258 = Bundle By Name(cluster=w558, "QueueAction"=DeviceQueue_Action."Measure_InSitu") -> (w557:T7)
        n259 = Enqueue Element(queue=w556, element=w557, error in (no error)=w554) -> (queue out=w555:refnum<queue>, error out=w545:errorcluster)  [unwired: 1 in, 1 out]
        n260 = Get Date/Time In Seconds() -> (seconds since 1Jan1904=w544:timestamp)
        n261 = Bundle By Name(cluster=w550, "QueueAction"=DataQueue_Action."Measure_InSituSpinCoating", "Time Stamp"=w544) -> (w551:T4)
        n262 = Enqueue Element(queue=w548, element=w551, error in (no error)=w545) -> (queue out=w547:refnum<queue>, error out=w546:errorcluster)  [unwired: 1 in, 1 out]
      }
      event "StartSpin_Button": Value Change {
        w566 = T7 {"QueueAction"=enum."TimeOut", "Numeric 1"=0.0, "Numeric 2"=0.0, "Boolean 1"=FALSE, "Boolean 2"=FALSE, "Spin Program"=[], "Spin Prg v07"=[], "Time Stamp"=timestamp(0 s since 1904-01-01), "TabControl"=enum."Measure"}  # Device Queue
        n263 = event-data() -> ()  [unwired: 1 in, 6 out]
        n264 = Bundle By Name(cluster=w566, "QueueAction"=DeviceQueue_Action."Arduino_StartProgram") -> (w565:T7)
        n265 = Enqueue Element(queue=w564, element=w565, error in (no error)=w560) -> (queue out=w562:refnum<queue>, error out=w561:errorcluster)  [unwired: 1 in, 1 out]
      }
      event "Milliseconds": Value Change {
        w575 = T7 {"QueueAction"=enum."TimeOut", "Numeric 1"=0.0, "Numeric 2"=0.0, "Boolean 1"=FALSE, "Boolean 2"=FALSE, "Spin Program"=[], "Spin Prg v07"=[], "Time Stamp"=timestamp(0 s since 1904-01-01), "TabControl"=enum."Measure"}  # Device Queue
        n266 = event-data() -> ()  [unwired: 1 in, 6 out]
        n267 = Bundle By Name(cluster=w575, "QueueAction"=DeviceQueue_Action."Arduino_SetMillis", "Numeric 1"="Milliseconds") -> (w571:T7)
        n268 = Enqueue Element(queue=w574, element=w571, error in (no error)=w572) -> (queue out=w570:refnum<queue>, error out=w569:errorcluster)  [unwired: 1 in, 1 out]
      }
      event "Speed": Value Change {
        w584 = T7 {"QueueAction"=enum."TimeOut", "Numeric 1"=0.0, "Numeric 2"=0.0, "Boolean 1"=FALSE, "Boolean 2"=FALSE, "Spin Program"=[], "Spin Prg v07"=[], "Time Stamp"=timestamp(0 s since 1904-01-01), "TabControl"=enum."Measure"}  # Device Queue
        n269 = event-data() -> ()  [unwired: 1 in, 6 out]
        n270 = Bundle By Name(cluster=w584, "QueueAction"=DeviceQueue_Action."Arduino_SetSpeed", "Numeric 1"="Speed") -> (w580:T7)
        n271 = Enqueue Element(queue=w583, element=w580, error in (no error)=w581) -> (queue out=w579:refnum<queue>, error out=w578:errorcluster)  [unwired: 1 in, 1 out]
      }
      event "Debug": Value Change {
        n272 = event-data() -> ()  [unwired: 1 in, 6 out]
        n273 = Select(t=u8 0, s="Debug", f=u8 2) -> (s? t:f=w585:u8)
        n274 = property on="Milliseconds" class="DigNum (strict)"("DisabledEnum"=w585) -> ()  [unwired: 2 in, 2 out]
        n275 = property on="Speed" class="DigNum (strict)"("DisabledEnum"=w585) -> ()  [unwired: 2 in, 2 out]
      }
      event "Frames for Spectrometer": Value Change {
        w598 = T7 {"QueueAction"=enum."TimeOut", "Numeric 1"=0.0, "Numeric 2"=0.0, "Boolean 1"=FALSE, "Boolean 2"=FALSE, "Spin Program"=[], "Spin Prg v07"=[], "Time Stamp"=timestamp(0 s since 1904-01-01), "TabControl"=enum."Measure"}  # Device Queue
        n276 = event-data() -> ("NewVal"=w592:dbl)  [unwired: 1 in, 5 out]
        n277 = Bundle By Name(cluster=w598, "QueueAction"=DeviceQueue_Action."Spectrometer_SetFrames", "Numeric 1"=w592) -> (w599:T7)
        n278 = Enqueue Element(queue=w596, element=w599) -> (queue out=w593:refnum<queue>)  [unwired: 2 in, 2 out]
      }
      event "Measure Spectrum": Value Change {
        w604 = T4 {"QueueAction"=enum."TimeOut", "Data"=[], "Data_Raw"=[], "Data_Dark"=[], "Data_Ref"=[], "Device Information"=[], "Numeric Control"=0.0, "Boolean"=FALSE, "Wavelength"=[], "Time"=[], "Time Stamp"=timestamp(0 s since 1904-01-01), "Numeric Control 2"=0.0, "TabControl"=enum."Measure"}  # DataQueue
        w610 = T7 {"QueueAction"=enum."TimeOut", "Numeric 1"=0.0, "Numeric 2"=0.0, "Boolean 1"=FALSE, "Boolean 2"=FALSE, "Spin Program"=[], "Spin Prg v07"=[], "Time Stamp"=timestamp(0 s since 1904-01-01), "TabControl"=enum."Measure"}  # Device Queue
        n279 = event-data() -> ()  [unwired: 1 in, 6 out]
        n280 = Bundle By Name(cluster=w610, "QueueAction"=DeviceQueue_Action."Measure_Spectrum") -> (w611:T7)
        n281 = Enqueue Element(queue=w608, element=w611) -> (queue out=w606:refnum<queue>)  [unwired: 2 in, 2 out]
        n282 = Get Date/Time In Seconds() -> (seconds since 1Jan1904=w605:timestamp)
        n283 = Bundle By Name(cluster=w604, "QueueAction"=DataQueue_Action."Measure_Spectrum", "Time Stamp"=w605) -> (w601:T4)
        n284 = Enqueue Element(queue=w602, element=w601) -> (queue out=w600:refnum<queue>)  [unwired: 2 in, 2 out]
      }
      event "Automatically \nadjust count": Value Change {
        n285 = event-data() -> ("NewVal"=w618:bool)  [unwired: 1 in, 5 out]
        n286 = Select(t=u8 2, s=w618, f=u8 0) -> (s? t:f=w612:u8)
        n287 = property on="Spectra Count" class="DigNum (strict)"("DisabledEnum"=w612) -> ()  [unwired: 2 in, 2 out]
      }
    }
  }
  n288 = while {
    shift-right: [w623] -> _
    shift-left: w8 -> [w627]
    shift-right: [w624] -> w10
    shift-left: w12 -> [w626]
    shift-right: [w621] -> w9
    shift-left: w7 -> [w622]
    shift-right: [w619] -> _
    shift-left: w11 -> [w620]
    stop <- w625 stop-if-true
    # "Consumer Devices"
    n289 = case shown="No Error" w627 {
      selector: w627 -> [w639 w1047]
      tunnel: w626 -> [w640 w1048]
      tunnel: [w636 _] -> w625
      tunnel: [w635 w1048] -> w624
      tunnel: [w633 w1044] -> w623
      tunnel: w622 -> [w631 w1042]
      tunnel: [w632 w1042] -> w621
      tunnel: w620 -> [w630 w1043]
      tunnel: [w629 w1043] -> w619
      frame No Error {
        n290 = Dequeue Element(queue=w640, error in (no error)=w639) -> (queue out=w638:refnum<queue>, element=w628:T7, error out=w634:errorcluster)  [unwired: 1 in, 1 out]
        n291 = Unbundle By Name(w628) -> ("QueueAction"=w637:T8)
        n292 = case shown="\"Measure_InSitu\"" w637 {
          tunnel: w638 -> [w644 w664 w670 w679 w729 w743 w753 w772 w779 w798 w799 w827 w844 w859 w869 w881 w893 w906 w926 w928 w935 w951 w964 w974 w1020 w1039]
          tunnel: [_ w666 _ _ _ _ _ _ _ _ _ _ _ _ _ _ _ _ _ _ _ _ _ _ _ _] -> w636
          tunnel: [w644 w649 w670 w678 w729 w743 w754 w772 w779 w798 w799 w827 w844 w859 w869 w881 w886 w906 w926 w928 w935 w951 w964 w974 w982 w1030] -> w635
          tunnel: w634 -> [w643 w648 w671 w690 w730 w742 w749 w775 w783 w795 w809 w825 w834 w850 w866 w877 w901 w910 w925 w930 w942 w952 w963 w967 w976 w1038]
          tunnel: [w643 w647 w669 w677 w724 w741 w747 w773 w780 w785 w803 w824 w831 w846 w864 w871 w885 w909 w921 w929 w936 w950 w959 w966 w983 w1029] -> w633
          tunnel: [w641 w646 w674 w675 w726 w738 w758 w771 w778 w789 w811 w828 w838 w853 w860 w873 w899 w908 w923 w934 w946 w948 w965 w969 w991 w1037] -> w632
          tunnel: w631 -> [w641 w646 w674 w676 w726 w739 w759 w771 w778 w790 w811 w828 w841 w856 w860 w875 w899 w908 w923 w934 w946 w948 w965 w970 w991 w1037]
          tunnel: w630 -> [w642 w645 w673 w687 w728 w740 w752 w770 w782 w791 w802 w821 w837 w852 w863 w870 w898 w907 w922 w933 w945 w947 w962 w968 w1023 w1036]
          tunnel: [w642 w645 w673 w681 w727 w740 w751 w768 w777 w791 w800 w822 w836 w851 w861 w870 w896 w907 w922 w933 w945 w947 w962 w968 w1023 w1036] -> w629
          tunnel: w628 -> [_ _ _ _ _ _ _ _ _ w797 w806 w829 _ _ w867 _ _ _ w920 _ w943 w949 _ _ _ _]
          frame "TimeOut", Default {
          }
          frame "Close_Program" {
            w665 = T7 {"QueueAction"=enum."TimeOut", "Numeric 1"=0.0, "Numeric 2"=0.0, "Boolean 1"=FALSE, "Boolean 2"=FALSE, "Spin Program"=[], "Spin Prg v07"=[], "Time Stamp"=timestamp(0 s since 1904-01-01), "TabControl"=enum."Measure"}  # Device Queue
            n293 = Bundle By Name(cluster=w665, "QueueAction"=DeviceQueue_Action."Spectrometer_Close") -> (w660:T7)
            n294 = Bundle By Name(cluster=w660, "QueueAction"=DeviceQueue_Action."Laser_Close") -> (w658:T7)
            n295 = Bundle By Name(cluster=w658, "QueueAction"=DeviceQueue_Action."Arduino_Close") -> (w652:T7)
            n296 = Enqueue Element(queue=w664, element=w660, error in (no error)=w648) -> (queue out=w662:refnum<queue>, error out=w657:errorcluster)  [unwired: 1 in, 1 out]
            n297 = Bundle By Name(cluster=w652, "QueueAction"=DeviceQueue_Action."Close_Program") -> (w650:T7)
            n298 = Enqueue Element(queue=w662, element=w658, error in (no error)=w657) -> (queue out=w656:refnum<queue>, error out=w655:errorcluster)  [unwired: 1 in, 1 out]
            n299 = Enqueue Element(queue=w656, element=w652, error in (no error)=w655) -> (queue out=w654:refnum<queue>, error out=w653:errorcluster)  [unwired: 1 in, 1 out]
            n300 = Enqueue Element(queue=w654, element=w650, error in (no error)=w653) -> (queue out=w649:refnum<queue>, error out=w647:errorcluster)  [unwired: 1 in, 1 out]
            n301 = First Call?() -> (First Call?: T/F=w667:bool)
            n302 = Not(x=w667) -> (.not. x?=w666:bool)
          }
          frame "Abort" {
            n303 = Unbundle By Name(w673) -> ("Port Arduino"=w672:refnum<visa-resource-name>)
            n304 = VISA Write(VISA resource name=w672, write buffer="abo", error in (no error)=w671) -> (error out=w669:errorcluster)  [unwired: 2 out]
          }
          frame "Spectrometer_Init" {
            n305 = call-dynamic "Init.vi"("error in (no error)"=w690, "Variant"=0, "Avantes in"=refnum<class "Avantes.lvclass"> refnum ("Avantes.lvclass")) -> ("error out"=w689:errorcluster, "Avantes out"=w688:refnum<class "Avantes.lvclass">)  [unwired: 7 in]
            n306 = call-dynamic "IsInit.vi"("error in (no error)"=w689, "Avantes in"=w688) -> ("error out"=w685:errorcluster, "Is Init?"=w684:bool, "Avantes out"=w686:refnum<class "Avantes.lvclass">)  [unwired: 7 in]
            n307 = property on="Spectromter" class="Bool (strict)"("Value"=w684) -> ()  [unwired: 2 in, 2 out]
            n308 = property on="Init_Spectrometer" class="Bool (strict)"("Value"=w684) -> ()  [unwired: 2 in, 2 out]
            n309 = call-dynamic "Set_ExposurePerFrame.vi"("error in (no error)"=w685, "Exposure per Frame"=1, "Avantes in"=w686) -> ("error out"=w680:errorcluster, "Avantes out"=w683:refnum<class "Avantes.lvclass">)  [unwired: 7 in]
            n310 = case shown="True" w684 {
              tunnel: w683 -> [_ w706]
              tunnel: w680 -> [w695 w704]
              tunnel: [refnum<class "Abstract_CCD.lvclass"> refnum ("Abstract_CCD.lvclass") w705] -> w682
              tunnel: w679 -> [w696 w721]
              tunnel: [w696 w710] -> w678
              tunnel: [w695 w709] -> w677
              tunnel: w676 -> [w694 w701]
              tunnel: [w694 w699] -> w675
              frame False {
              }
              frame True {
                w707 = T4 {"QueueAction"=enum."TimeOut", "Data"=[], "Data_Raw"=[], "Data_Dark"=[], "Data_Ref"=[], "Device Information"=[], "Numeric Control"=0.0, "Boolean"=FALSE, "Wavelength"=[], "Time"=[], "Time Stamp"=timestamp(0 s since 1904-01-01), "Numeric Control 2"=0.0, "TabControl"=enum."Measure"}  # DataQueue
                w722 = T7 {"QueueAction"=enum."TimeOut", "Numeric 1"=0.0, "Numeric 2"=0.0, "Boolean 1"=FALSE, "Boolean 2"=FALSE, "Spin Program"=[], "Spin Prg v07"=[], "Time Stamp"=timestamp(0 s since 1904-01-01), "TabControl"=enum."Measure"}  # Device Queue
                n311 = call-dynamic "Get_WavelengthAxis.vi"("error in (no error)"=w704, "Avantes in"=w706) -> ("error out"=w703:errorcluster, "lambda"=w698:dbl[unit][], "Avantes out"=w705:refnum<class "Avantes.lvclass">)  [unwired: 7 in]
                n312 = property on="Calculate Frames" class="Bool (strict)"() -> ("Value"=w714:bool)  [unwired: 2 in, 2 out]
                n313 = property on="Integration Time" class="DigNum (strict)"() -> ("Value"=w719:dbl[unit])  [unwired: 2 in, 2 out]
                n314 = Unbundle(w703) -> ("status"=w702:bool)  [unwired: 2 out]
                n315 = node(w719) -> (w718:dbl)
                n316 = Bundle By Name(cluster=w722, "QueueAction"=DeviceQueue_Action."Spectrometer_SetIntegrationTime", "Numeric 1"=w718, "Boolean 1"=w714) -> (w716:T7)
                n317 = property on="Frames" class="DigNum (strict)"() -> ("Value"=w713:i32)  [unwired: 2 in, 2 out]
                n318 = property on="Error_Spectromter" class="Bool (strict)"("Value"=w702) -> ()  [unwired: 2 in, 2 out]
                n319 = Enqueue Element(queue=w721, element=w716, error in (no error)=w704) -> (queue out=w717:refnum<queue>, error out=w711:errorcluster)  [unwired: 1 in, 1 out]
                n320 = Bundle By Name(cluster=w716, "QueueAction"=DeviceQueue_Action."Spectrometer_SetFrames", "Numeric 1"=w713) -> (w712:T7)
                n321 = Bundle By Name(cluster=w707, "QueueAction"=DataQueue_Action."Set_Wavelength", "Wavelength"=w698) -> (w708:T4)
                n322 = Enqueue Element(queue=w701, element=w708) -> (queue out=w699:refnum<queue>)  [unwired: 2 in, 2 out]
                n323 = Enqueue Element(queue=w717, element=w712, error in (no error)=w711) -> (queue out=w710:refnum<queue>, error out=w709:errorcluster)  [unwired: 1 in, 1 out]
              }
            }
            n324 = Bundle By Name(cluster=w687, "Abstract_CCD.lvclass"=w682) -> (w681:T3)
          }
          frame "Spectrometer_Close" {
            n325 = property on="Spectromter" class="Bool (strict)"("Value"=FALSE ("Spectromter")) -> ()  [unwired: 2 in, 2 out]
            n326 = Unbundle By Name(w728) -> ("Abstract_CCD.lvclass"=w731:refnum<class "Abstract_CCD.lvclass">)
            n327 = flat-sequence {
              tunnel: [refnum<class "Abstract_CCD.lvclass"> refnum ("Abstract_CCD.lvclass")] -> w725
              tunnel: w724 -> [_]
              frame #0 {
              }
            }
            n328 = call-dynamic "Close.vi"("error in (no error)"=w730, "Abstract_CCD in"=w731) -> ("error out"=w724:errorcluster)  [unwired: 8 in, 1 out]
            n329 = Bundle By Name(cluster=w728, "Abstract_CCD.lvclass"=w725) -> (w727:T3)
          }
          frame "Spectrometer_Measure" {
            w745 = T4 {"QueueAction"=enum."TimeOut", "Data"=[], "Data_Raw"=[], "Data_Dark"=[], "Data_Ref"=[], "Device Information"=[], "Numeric Control"=0.0, "Boolean"=FALSE, "Wavelength"=[], "Time"=[], "Time Stamp"=timestamp(0 s since 1904-01-01), "Numeric Control 2"=0.0, "TabControl"=enum."Measure"}  # DataQueue
            n330 = Unbundle By Name(w740) -> ("Abstract_CCD.lvclass"=w744:refnum<class "Abstract_CCD.lvclass">)
            n331 = call-dynamic "Measure.vi"("error in (no error)"=w742, "Abstract_CCD in"=w744) -> ("error out"=w741:errorcluster, "Data Raw"=w735:T11, "Data"=w736:T11, "Darkspec"=w734:T11, "Time"=w733:dbl[])  [unwired: 3 in, 2 out]
            n332 = Bundle By Name(cluster=w745, "QueueAction"=DataQueue_Action."Spectrometer_Measure", "Data"=w736, "Data_Raw"=w735, "Data_Dark"=w734, "Time"=w733) -> (w746:T4)
            n333 = Enqueue Element(queue=w739, element=w746) -> (queue out=w738:refnum<queue>)  [unwired: 2 in, 2 out]
          }
          frame "Spectrometer_Preview" {
            w760 = T4 {"QueueAction"=enum."TimeOut", "Data"=[], "Data_Raw"=[], "Data_Dark"=[], "Data_Ref"=[], "Device Information"=[], "Numeric Control"=0.0, "Boolean"=FALSE, "Wavelength"=[], "Time"=[], "Time Stamp"=timestamp(0 s since 1904-01-01), "Numeric Control 2"=0.0, "TabControl"=enum."Measure"}  # DataQueue
            n334 = Unbundle By Name(w752) -> ("Abstract_CCD.lvclass"=w750:refnum<class "Abstract_CCD.lvclass">)
            n335 = call-dynamic "Measure.vi"("error in (no error)"=w749, "Abstract_CCD in"=w750) -> ("error out"=w747:errorcluster, "Data Raw"=w757:T11, "Abstract_CCD out"=w748:refnum<class "Abstract_CCD.lvclass">)  [unwired: 3 in, 4 out]
            n336 = property on="Preview" class="Bool (strict)"(error in=w747) -> ("Value"=w755:bool)  [unwired: 1 in, 2 out]
            n337 = case shown="True" w755 {
              tunnel: [w762 w764] -> w754
              tunnel: w753 -> [w762 w763]
              frame False {
              }
              frame True {
                w766 = T7 {"QueueAction"=enum."TimeOut", "Numeric 1"=0.0, "Numeric 2"=0.0, "Boolean 1"=FALSE, "Boolean 2"=FALSE, "Spin Program"=[], "Spin Prg v07"=[], "Time Stamp"=timestamp(0 s since 1904-01-01), "TabControl"=enum."Measure"}  # Device Queue
                n338 = Bundle By Name(cluster=w766, "QueueAction"=DeviceQueue_Action."Spectrometer_Preview") -> (w765:T7)
                n339 = Enqueue Element(queue=w763, element=w765) -> (queue out=w764:refnum<queue>)  [unwired: 2 in, 2 out]
              }
            }
            n340 = Bundle By Name(cluster=w760, "Data_Raw"=w757, "QueueAction"=DataQueue_Action."Spectrometer_Preview") -> (w761:T4)
            n341 = Enqueue Element(queue=w759, element=w761) -> (queue out=w758:refnum<queue>)  [unwired: 2 in, 2 out]
            n342 = Bundle By Name(cluster=w752, "Abstract_CCD.lvclass"=w748) -> (w751:T3)
          }
          frame "Spectrometer_StartMeasurement" {
            n343 = Unbundle By Name(w770) -> ("Abstract_CCD.lvclass"=w774:refnum<class "Abstract_CCD.lvclass">)
            n344 = call-dynamic "StartMeasure.vi"("error in (no error)"=w775, "Frames"=-1, "Abstract_CCD in"=w774) -> ("error out"=w773:errorcluster, "Abstract_CCD out"=w769:refnum<class "Abstract_CCD.lvclass">)  [unwired: 7 in]
            n345 = Bundle By Name(cluster=w770, "Abstract_CCD.lvclass"=w769) -> (w768:T3)
          }
          frame "Spectrometer_StopMeasurement" {
            n346 = Unbundle By Name(w782) -> ("Abstract_CCD.lvclass"=w784:refnum<class "Abstract_CCD.lvclass">)
            n347 = call-dynamic "StopMeasurement.vi"("error in (no error)"=w783, "Abstract_CCD in"=w784) -> ("error out"=w780:errorcluster, "Abstract_CCD out"=w781:refnum<class "Abstract_CCD.lvclass">)  [unwired: 8 in]
            n348 = Bundle By Name(cluster=w782, "Abstract_CCD.lvclass"=w781) -> (w777:T3)
          }
          frame "Spectrometer_GetData" {
            w794 = T4 {"QueueAction"=enum."TimeOut", "Data"=[], "Data_Raw"=[], "Data_Dark"=[], "Data_Ref"=[], "Device Information"=[], "Numeric Control"=0.0, "Boolean"=FALSE, "Wavelength"=[], "Time"=[], "Time Stamp"=timestamp(0 s since 1904-01-01), "Numeric Control 2"=0.0, "TabControl"=enum."Measure"}  # DataQueue
            n349 = Unbundle By Name(w791) -> ("Abstract_CCD.lvclass"=w796:refnum<class "Abstract_CCD.lvclass">)
            n350 = Unbundle By Name(w797) -> ("Numeric 1"=w788:dbl)
            n351 = call-dynamic "Measure_GetData.vi"("error in (no error)"=w795, "SpectraCount"=w788, "Abstract_CCD in"=w796) -> ("error out"=w785:errorcluster, "Data_Raw"=w787:T11, "Time"=w786:dbl[])  [unwired: 5 in, 1 out]
            n352 = Bundle By Name(cluster=w794, "QueueAction"=DataQueue_Action."Spectrometer_Measure", "Data_Raw"=w787, "Time"=w786) -> (w793:T4)
            n353 = Enqueue Element(queue=w790, element=w793) -> (queue out=w789:refnum<queue>)  [unwired: 2 in, 2 out]
          }
          frame "Spectrometer_SetIntegrationTime" {
            n354 = Unbundle By Name(w806) -> ("Numeric 1"=w808:dbl)
            n355 = Unbundle By Name(w802) -> ("Abstract_CCD.lvclass"=w810:refnum<class "Abstract_CCD.lvclass">)
            n356 = Unbundle By Name(w806) -> ("Boolean 1"=w805:bool)
            n357 = node(w808) -> (w807:dbl[unit])
            n358 = call-dynamic "Set_ExposureTime.vi"("error in (no error)"=w809, "Exposure Time"=w807, "Abstract_CCD in"=w810) -> ("error out"=w813:errorcluster, "Abstract_CCD out"=w812:refnum<class "Abstract_CCD.lvclass">)  [unwired: 7 in]
            n359 = call-dynamic "Get_FrameRate.vi"("error in (no error)"=w813, "Abstract_CCD in"=w812) -> ("error out"=w803:errorcluster, "Frame Rate"=w804:dbl[unit], "Abstract_CCD out"=w801:refnum<class "Abstract_CCD.lvclass">)  [unwired: 7 in]
            "Frame Rate" <- w804
            n360 = Bundle By Name(cluster=w802, "Abstract_CCD.lvclass"=w801) -> (w800:T3)
            n361 = case shown="True" w805 {
              tunnel: w804 -> [_ w816]
              frame False {
              }
              frame True {
                n362 = property on="Program Spin Coater\nSpeed (rpm)          Time (s)" class="Arr (strict)"() -> ("Value"=w819:dbl[][])  [unwired: 2 in, 2 out]
                n363 = property on="Seconds to Spin Start" class="DigNum (strict)"() -> ("Value"=w818:dbl[unit])  [unwired: 2 in, 2 out]
                n364 = property on="Seconds after Spin Stop" class="DigNum (strict)"() -> ("Value"=w817:dbl[unit])  [unwired: 2 in, 2 out]
                n365 = call "CalculateFrames.vi"("Program Spin Coater\nSpeed (rpm)          Time (s)"=w819, "Seconds End"=w817, "Seconds Start"=w818, "Frame Rate"=w816) -> ("Time"=w815:dbl, "Frames"=w814:i32)  [unwired: 6 in]
                n366 = property on="Overall Time" class="DigNum (strict)"("Value"=w815) -> ()  [unwired: 2 in, 2 out]
                n367 = property on="Frames" class="DigNum (strict)"("Value"=w814) -> ()  [unwired: 2 in, 2 out]
              }
            }
          }
          frame "Spectrometer_SetFrames" {
            n368 = Unbundle By Name(w821) -> ("Abstract_CCD.lvclass"=w826:refnum<class "Abstract_CCD.lvclass">)
            n369 = Unbundle By Name(w829) -> ("Numeric 1"=w823:dbl)
            n370 = call-dynamic "Set_Frames.vi"("error in (no error)"=w825, "Frames"=w823, "Abstract_CCD in"=w826) -> ("error out"=w824:errorcluster, "Abstract_CCD out"=w820:refnum<class "Abstract_CCD.lvclass">)  [unwired: 7 in]
            n371 = Bundle By Name(cluster=w821, "Abstract_CCD.lvclass"=w820) -> (w822:T3)
          }
          frame "Spectrometer_SetDarkspec" {
            w842 = T4 {"QueueAction"=enum."TimeOut", "Data"=[], "Data_Raw"=[], "Data_Dark"=[], "Data_Ref"=[], "Device Information"=[], "Numeric Control"=0.0, "Boolean"=FALSE, "Wavelength"=[], "Time"=[], "Time Stamp"=timestamp(0 s since 1904-01-01), "Numeric Control 2"=0.0, "TabControl"=enum."Measure"}  # DataQueue
            n372 = Unbundle By Name(w837) -> ("Abstract_CCD.lvclass"=w835:refnum<class "Abstract_CCD.lvclass">)
            n373 = call-dynamic "Measure.vi"("error in (no error)"=w834, "Abstract_CCD in"=w835) -> ("error out"=w832:errorcluster, "Data Raw"=w839:T11, "Abstract_CCD out"=w833:refnum<class "Abstract_CCD.lvclass">)  [unwired: 3 in, 4 out]
            n374 = Bundle By Name(cluster=w842, "QueueAction"=DataQueue_Action."Set_Dark", "Data_Dark"=w839) -> (w843:T4)
            n375 = Enqueue Element(queue=w841, element=w843) -> (queue out=w838:refnum<queue>)  [unwired: 2 in, 2 out]
            n376 = Bundle By Name(cluster=w837, "Abstract_CCD.lvclass"=w833) -> (w836:T3)
            n377 = property on="Record_Darkspec" class="Bool (strict)"(error in=w832, "Value"=FALSE ("Record_Darkspec")) -> (error out=w831:errorcluster)  [unwired: 1 in, 1 out]
          }
          frame "Spectrometer_SetReference" {
            w857 = T4 {"QueueAction"=enum."TimeOut", "Data"=[], "Data_Raw"=[], "Data_Dark"=[], "Data_Ref"=[], "Device Information"=[], "Numeric Control"=0.0, "Boolean"=FALSE, "Wavelength"=[], "Time"=[], "Time Stamp"=timestamp(0 s since 1904-01-01), "Numeric Control 2"=0.0, "TabControl"=enum."Measure"}  # DataQueue
            n378 = Unbundle By Name(w852) -> ("Abstract_CCD.lvclass"=w849:refnum<class "Abstract_CCD.lvclass">)
            n379 = call-dynamic "Measure.vi"("error in (no error)"=w850, "Abstract_CCD in"=w849) -> ("error out"=w847:errorcluster, "Data Raw"=w854:T11, "Abstract_CCD out"=w848:refnum<class "Abstract_CCD.lvclass">)  [unwired: 3 in, 4 out]
            n380 = Bundle By Name(cluster=w857, "QueueAction"=DataQueue_Action."Set_Ref", "Data_Ref"=w854) -> (w858:T4)
            n381 = Enqueue Element(queue=w856, element=w858) -> (queue out=w853:refnum<queue>)  [unwired: 2 in, 2 out]
            n382 = Bundle By Name(cluster=w852, "Abstract_CCD.lvclass"=w848) -> (w851:T3)
            n383 = property on="Record RefSpec" class="Bool (strict)"(error in=w847, "Value"=FALSE ("Record RefSpec")) -> (error out=w846:errorcluster)  [unwired: 1 in, 1 out]
          }
          frame "Spectrometer_SetTriggerMode" {
            n384 = Unbundle By Name(w863) -> ("Abstract_CCD.lvclass"=w868:refnum<class "Abstract_CCD.lvclass">)
            n385 = Unbundle By Name(w867) -> ("Numeric 1"=w865:dbl)
            n386 = call-dynamic "Set_TriggerMode.vi"("error in (no error)"=w866, "Trigger Mode"=w865, "Abstract_CCD in"=w868) -> ("error out"=w864:errorcluster, "Abstract_CCD out"=w862:refnum<class "Abstract_CCD.lvclass">)  [unwired: 7 in]
            n387 = Bundle By Name(cluster=w863, "Abstract_CCD.lvclass"=w862) -> (w861:T3)
          }
          frame "Spectrometer_DeviceInformation" {
            w876 = T4 {"QueueAction"=enum."TimeOut", "Data"=[], "Data_Raw"=[], "Data_Dark"=[], "Data_Ref"=[], "Device Information"=[], "Numeric Control"=0.0, "Boolean"=FALSE, "Wavelength"=[], "Time"=[], "Time Stamp"=timestamp(0 s since 1904-01-01), "Numeric Control 2"=0.0, "TabControl"=enum."Measure"}  # DataQueue
            n388 = Unbundle By Name(w870) -> ("Abstract_CCD.lvclass"=w878:refnum<class "Abstract_CCD.lvclass">)
            n389 = call-dynamic "Get_DeviceInformation.vi"("error in (no error)"=w877, "Abstract_CCD in"=w878) -> ("error out"=w872:errorcluster, "Array"=w879:string[])  [unwired: 7 in, 1 out]
            n390 = Bundle By Name(cluster=w876, "QueueAction"=DataQueue_Action."Transfer_Settings", "Device Information"=w879) -> (w874:T4)
            n391 = Enqueue Element(queue=w875, element=w874, error in (no error)=w872) -> (queue out=w873:refnum<queue>, error out=w871:errorcluster)  [unwired: 1 in, 1 out]
          }
          frame "Arduino_Init" {
            w895 = T7 {"QueueAction"=enum."TimeOut", "Numeric 1"=0.0, "Numeric 2"=0.0, "Boolean 1"=FALSE, "Boolean 2"=FALSE, "Spin Program"=[], "Spin Prg v07"=[], "Time Stamp"=timestamp(0 s since 1904-01-01), "TabControl"=enum."Measure"}  # Device Queue
            n392 = call-poly "VISA Configure Serial Port"("VISA resource name"="Port Arduino", "baud rate (9600)"=u32 115200, "error in (no error)"=w901) -> ("VISA resource name out"=w897:refnum<visa-resource-name>, "error out"=w884:errorcluster)  [unwired: 11 in]
            n393 = Unbundle(w884) -> ("status"=w883:bool)  [unwired: 2 out]
            n394 = Not(x=w883) -> (.not. x?=w882:bool)
            n395 = property on="Arduino" class="Bool (strict)"("Value"=w882) -> ()  [unwired: 2 in, 2 out]
            n396 = property on="Program Spin Coater\nSpeed (rpm)          Time (s)" class="Arr (strict)"() -> ("Value"=w890:dbl[][])  [unwired: 2 in, 2 out]
            n397 = Bundle By Name(cluster=w895, "QueueAction"=DeviceQueue_Action."Arduino_LoadProgram", "Spin Program"=dbl[][] []) -> (w891:T7)
            n398 = Enqueue Element(queue=w893, element=w891, error in (no error)=w884) -> (queue out=w889:refnum<queue>, error out=w888:errorcluster)  [unwired: 1 in, 1 out]
            n399 = Bundle By Name(cluster=w891, "Spin Program"=w890) -> (w887:T7)
            n400 = Bundle By Name(cluster=w898, "Port Arduino"=w897) -> (w896:T3)
            n401 = Enqueue Element(queue=w889, element=w887, error in (no error)=w888) -> (queue out=w886:refnum<queue>, error out=w885:errorcluster)  [unwired: 1 in, 1 out]
          }
          frame "Arduino_Close" {
            n402 = property on="Arduino" class="Bool (strict)"() -> (error out=w904:errorcluster, "Value"=w903:bool)  [unwired: 2 in, 1 out]
            n403 = Unbundle By Name(w907) -> ("Port Arduino"=w911:refnum<visa-resource-name>)
            n404 = property on="Arduino" class="Bool (strict)"(error in=w904, "Value"=FALSE ("Arduino")) -> ()  [unwired: 1 in, 2 out]
            n405 = case shown="False" w903 {
              tunnel: w911 -> [_ w915]
              tunnel: w910 -> [w912 w914]
              tunnel: [w912 w913] -> w909
              frame False {
              }
              frame True {
                n406 = VISA Close(VISA resource name=w915, error in (no error)=w914) -> (error out=w913:errorcluster)
              }
            }
          }
          frame "Arduino_LoadProgram" {
            n407 = Unbundle By Name(w920) -> ("Spin Program"=w919:dbl[][], "Numeric 1"=w917:dbl)
            n408 = Unbundle By Name(w922) -> ("Port Arduino"=w924:refnum<visa-resource-name>)
            n409 = node(w917) -> (w916:dbl[unit])
            n410 = call "SpinCoaterArray2String_v02.vi"("Time Start"=w916, "Program Spin Coater\nSpeed (rpm)          Time (s)"=w919) -> ("remote control String"=w918:string)  [unwired: 3 in]
            n411 = VISA Write(VISA resource name=w924, write buffer=w918, error in (no error)=w925) -> (error out=w921:errorcluster)  [unwired: 2 out]
          }
          frame "Arduino_StartProgram" {
            n412 = Unbundle By Name(w933) -> ("Port Arduino"=w932:refnum<visa-resource-name>)
            n413 = VISA Write(VISA resource name=w932, write buffer="run", error in (no error)=w930) -> (error out=w929:errorcluster)  [unwired: 2 out]
            n414 = property on="Action" class="Str"("Value"="Measuring" ("Action")) -> ()  [unwired: 2 in, 2 out]
          }
          frame "Arduino_SetSpeed" {
            n415 = Unbundle By Name(w943) -> ("Numeric 1"=w941:dbl)
            n416 = Unbundle By Name(w945) -> ("Port Arduino"=w944:refnum<visa-resource-name>)
            n417 = To Unsigned Long Integer(number=w941) -> (unsigned 32bit integer=w940:u32)
            n418 = Number To Decimal String(number=w940) -> (decimal integer string=w939:string)  [unwired: 1 in]
            n419 = Concatenate Strings("!spe" ("string"), w939) -> (w937:string)
            n420 = VISA Write(VISA resource name=w944, write buffer=w937, error in (no error)=w942) -> (error out=w936:errorcluster)  [unwired: 2 out]
          }
          frame "Arduino_SetMillis" {
            n421 = Unbundle By Name(w949) -> ("Numeric 1"=w957:dbl)
            n422 = Unbundle By Name(w947) -> ("Port Arduino"=w958:refnum<visa-resource-name>)
            n423 = To Unsigned Long Integer(number=w957) -> (unsigned 32bit integer=w956:u32)
            n424 = Number To Decimal String(number=w956) -> (decimal integer string=w955:string)  [unwired: 1 in]
            n425 = Concatenate Strings("!mil" ("string"), w955) -> (w953:string)
            n426 = VISA Write(VISA resource name=w958, write buffer=w953, error in (no error)=w952) -> (error out=w950:errorcluster)  [unwired: 2 out]
          }
          frame "Arduino_StopSpin" {
            n427 = Unbundle By Name(w962) -> ("Port Arduino"=w961:refnum<visa-resource-name>)
            n428 = VISA Write(VISA resource name=w961, write buffer="abo", error in (no error)=w963) -> (error out=w959:errorcluster)  [unwired: 2 out]
          }
          frame "Measure_Stop" {
            w972 = T4 {"QueueAction"=enum."TimeOut", "Data"=[], "Data_Raw"=[], "Data_Dark"=[], "Data_Ref"=[], "Device Information"=[], "Numeric Control"=0.0, "Boolean"=FALSE, "Wavelength"=[], "Time"=[], "Time Stamp"=timestamp(0 s since 1904-01-01), "Numeric Control 2"=0.0, "TabControl"=enum."Measure"}  # DataQueue
            n429 = Bundle By Name(cluster=w972, "QueueAction"=DataQueue_Action."Stop_Measurement") -> (w973:T4)
            n430 = Enqueue Element(queue=w970, element=w973, error in (no error)=w967) -> (queue out=w969:refnum<queue>, error out=w966:errorcluster)  [unwired: 1 in, 1 out]
          }
          frame "Measure_InSitu" {
            w1014 = T7 {"QueueAction"=enum."TimeOut", "Numeric 1"=0.0, "Numeric 2"=0.0, "Boolean 1"=FALSE, "Boolean 2"=FALSE, "Spin Program"=[], "Spin Prg v07"=[], "Time Stamp"=timestamp(0 s since 1904-01-01), "TabControl"=enum."Measure"}  # Device Queue
            w1021 = T7 {"QueueAction"=enum."TimeOut", "Numeric 1"=0.0, "Numeric 2"=0.0, "Boolean 1"=FALSE, "Boolean 2"=FALSE, "Spin Program"=[], "Spin Prg v07"=[], "Time Stamp"=timestamp(0 s since 1904-01-01), "TabControl"=enum."Measure"}  # Device Queue
            n431 = Bundle By Name(cluster=w1021, "QueueAction"=DeviceQueue_Action."Spectrometer_SetTriggerMode", "Numeric 1"=1.0) -> (w1019:T7)
            n432 = Bundle By Name(cluster=w1014, "QueueAction"=DeviceQueue_Action."Spectrometer_DeviceInformation") -> (w1011:T7)
            n433 = Bundle By Name(cluster=w1011, "QueueAction"=DeviceQueue_Action."Spectrometer_StartMeasurement") -> (w1007:T7)
            n434 = Enqueue Element(queue=w1020, element=w1019, error in (no error)=w976) -> (queue out=w1016:refnum<queue>, error out=w1017:errorcluster)  [unwired: 1 in, 1 out]
            n435 = property on="Frames" class="DigNum (strict)"() -> ("Value"=w977:i32)  [unwired: 2 in, 2 out]
            n436 = Bundle By Name(cluster=w1007, "QueueAction"=DeviceQueue_Action."Arduino_StartProgram") -> (w1002:T7)
            n437 = Enqueue Element(queue=w1016, element=w1011, error in (no error)=w1017) -> (queue out=w1013:refnum<queue>, error out=w1012:errorcluster)  [unwired: 1 in, 1 out]
            n438 = Bundle By Name(cluster=w1002, "QueueAction"=DeviceQueue_Action."Spectrometer_GetData", "Numeric 1"="Dividider Get Spectra") -> (w997:T7)
            n439 = Divide(x=w977, y="Dividider Get Spectra") -> (x/y=w1009:dbl)
            n440 = Round Toward +Infinity(x=w1009) -> (ceil(x): smallest int >= x=w1008:dbl)
            n441 = Enqueue Element(queue=w1013, element=w1007, error in (no error)=w1012) -> (queue out=w1006:refnum<queue>, error out=w1005:errorcluster)  [unwired: 1 in, 1 out]
            n442 = Enqueue Element(queue=w1006, element=w1002, error in (no error)=w1005) -> (queue out=w1003:refnum<queue>, error out=w1000:errorcluster)  [unwired: 1 in, 1 out]
            n443 = for {
              N: w1008 -> [_]
              shift-right: [w1024] -> w999
              shift-left: w1003 -> [w1028]
              tunnel: w997 -> [w1025]
              shift-right: [w1026] -> w998
              shift-left: w1000 -> [w1027]
              n444 = Enqueue Element(queue=w1028, element=w1025, error in (no error)=w1027) -> (queue out=w1024:refnum<queue>, error out=w1026:errorcluster)  [unwired: 1 in, 1 out]
            }
            n445 = Bundle By Name(cluster=w997, "QueueAction"=DeviceQueue_Action."Spectrometer_StopMeasurement") -> (w993:T7)
            n446 = property on="Frames for Spectrometer" class="DigNum (strict)"() -> ("Value"=w979:dbl)  [unwired: 2 in, 2 out]
            n447 = Bundle By Name(cluster=w993, "QueueAction"=DeviceQueue_Action."Measure_Stop") -> (w986:T7)
            n448 = Enqueue Element(queue=w999, element=w993, error in (no error)=w998) -> (queue out=w994:refnum<queue>, error out=w995:errorcluster)  [unwired: 1 in, 1 out]
            n449 = Bundle By Name(cluster=w986, "QueueAction"=DeviceQueue_Action."Spectrometer_SetTriggerMode", "Numeric 1"=0.0) -> (w981:T7)
            n450 = Enqueue Element(queue=w994, element=w986, error in (no error)=w995) -> (queue out=w989:refnum<queue>, error out=w990:errorcluster)  [unwired: 1 in, 1 out]
            n451 = Bundle By Name(cluster=w981, "QueueAction"=DeviceQueue_Action."Spectrometer_SetFrames", "Numeric 1"=w979) -> (w978:T7)
            n452 = Enqueue Element(queue=w989, element=w981, error in (no error)=w990) -> (queue out=w988:refnum<queue>, error out=w987:errorcluster)  [unwired: 1 in, 1 out]
            n453 = Enqueue Element(queue=w988, element=w978, error in (no error)=w987) -> (queue out=w982:refnum<queue>, error out=w983:errorcluster)  [unwired: 1 in, 1 out]
          }
          frame "Measure_Spectrum" {
            w1041 = T7 {"QueueAction"=enum."TimeOut", "Numeric 1"=0.0, "Numeric 2"=0.0, "Boolean 1"=FALSE, "Boolean 2"=FALSE, "Spin Program"=[], "Spin Prg v07"=[], "Time Stamp"=timestamp(0 s since 1904-01-01), "TabControl"=enum."Measure"}  # Device Queue
            n454 = Bundle By Name(cluster=w1041, "QueueAction"=DeviceQueue_Action."Spectrometer_Measure") -> (w1033:T7)
            n455 = Bundle By Name(cluster=w1033, "QueueAction"=DeviceQueue_Action."Measure_Stop") -> (w1031:T7)
            n456 = Enqueue Element(queue=w1039, element=w1033, error in (no error)=w1038) -> (queue out=w1034:refnum<queue>, error out=w1035:errorcluster)  [unwired: 1 in, 1 out]
            n457 = Enqueue Element(queue=w1034, element=w1031, error in (no error)=w1035) -> (queue out=w1030:refnum<queue>, error out=w1029:errorcluster)  [unwired: 1 in, 1 out]
          }
        }
      }
      frame Error {
        w1046 = T16 4 items=["no dialog", "OK message", "continue or stop message", "OK message + warnings", "continue/stop + warnings"] ("type of dialog (OK msg:1)")
        n458 = call <vilib>:"General Error Handler.vi"("type of dialog (OK msg:1)"=w1046, "error in (no error)"=w1047) -> ("error out"=w1045:errorcluster)  [unwired: 9 in, 4 out]
        n459 = call <vilib>:"Clear Errors.vi"("error in (no error)"=w1045) -> ("error out"=w1044:errorcluster)  [unwired: 5 in, 1 out]
      }
    }
  }
  n460 = disable-structure shown="Enabled" {
    frame Disabled {
      w1050 = T7 {"QueueAction"=enum."TimeOut", "Numeric 1"=0.0, "Numeric 2"=0.0, "Boolean 1"=FALSE, "Boolean 2"=FALSE, "Spin Program"=[], "Spin Prg v07"=[], "Time Stamp"=timestamp(0 s since 1904-01-01), "TabControl"=enum."Measure"}  # Device Queue
      n461 = Bundle By Name(cluster=w1050, "QueueAction"=DeviceQueue_Action."Arduino_SetSpeed") -> (w1049:T7)  [unwired: 1 in]
      n462 = Enqueue Element(element=w1049) -> ()  [unwired: 3 in, 3 out]
    }
    frame Enabled {
    }
  }
  n463 = Release Queue(queue=w9) -> ()  [unwired: 2 in, 3 out]
  n464 = Release Queue(queue=w10) -> ()  [unwired: 2 in, 3 out]
